vi "slow_control_2_10.vi"() -> ()   [LabVIEW 2018]
uses:
  4623b864-5764-45c6-9cb2-3e18237880ca.vi
  fa57f61f-0bb9-49ac-92eb-fcb40add4dbb.vi
  499f9cf5-7b15-41ea-951a-8da9be12721d.vi
  <vilib>/DAQmx/read.llb/DAQmx Read (Analog 1D DBL NChan 1Samp).vi
  ffb0d1b3-ef19-4e2e-b36e-7277177ef4b3.vi
  9a1acc8a-69db-4048-9e4c-bb07d66d2422.vi
  <vilib>/DAQmx/create/channels.llb/DAQmx Create Channel (AI-Voltage-Basic).vi
  <vilib>/DAQmx/create/channels.llb/DAQmx Create Channel (AI-Current-Basic).vi
  <vilib>/DAQmx/create/channels.llb/DAQmx Create Channel (AI-Temperature-RTD).vi
  <vilib>/DAQmx/miscellaneous.llb/DAQmx Fill In Error Info.vi
  <vilib>/Utility/file.llb/Read Delimited Spreadsheet (string).vi
  <instrlib>/Lake Shore 335/Lake Shore 335.lvlib
  <instrlib>/CAEN PSM/CAEN PSM.lvlib
  <resource>/objmgr/daqmx.rc
panel:
  out "Heater":dbl
  out "Coldhead":dbl
  out "Cycle number":i32
  out "Alarm state":bool
  out "Timestamp last \nmeasured (UPS)":timestamp
  out "Auto-clear":bool
  in  "Auto-clear data?":bool
  in  "Clear data":bool
  in  "Clear data every N cycles":dbl
  in  "N samples":i32=30
  out "Average Flow (SLPM)":dbl caption="Flow (SLPM)"
  out "CAEN Ch. Names":string[](array[string])
  in  "Cycles to execute":dbl=5.0 format="%#_13g"
  out "Detector Pressure":dbl
  in  "N samples":i32=20
  in  "Allows tabs on \nfront panel":T1(tab)
  in  "Specify up to six temperature sensors inside \nthe detector, separated with a comma.\nNumbers only, single commas!":string="10,11,12,13,14,15"
  out "Valid example:":string="11,12, 13, 15 ,14 "
  in  "Anode ch.":enum16{"1", "2", "3", "4"}(ring)=enum."3"
  in  "CAEN unit selector":enum16{"CAEN 1", "CAEN 2"}(ring)
  in  "Multipliers":dbl[](array[numeric])=[1.0, 1.0, 1.0, 1.0, 1.0, 1.0, 1.0, 1.0]
  in  "Offsets\nsubtracted":dbl[](array[numeric])=[0.0, 0.0, 0.0, 0.0, 0.0, 0.0, 0.0, 0.0]
  in  "Channel Names (9207, ai8:15)":string[](array[string])=["i0", "i1", "i2", "i3", "i4", "i5", "i6", "i7"] caption="\"Other\""
  in  "Flow meter input:":u16(ring)=3 items=["v0", "v1", "v2", "v3", "v4", "v5", "v6", "v7"]
  in  "Detector pressure input:":u16(ring) items=["v0", "v1", "v2", "v3", "v4", "v5", "v6", "v7"]
  in  "Channel Names (9207, ai0:7)":string[](array[string])=["v0", "v1", "v2", "v3", "v4", "v5", "v6", "v7"] caption="\"Other\""
  in  "Multipliers":dbl[](array[numeric])=[1.0, 1.0, 1.0, 1.0, 1.0, 1.0, 1.0, 1.0]
  in  "Offsets\nsubtracted":dbl[](array[numeric])=[0.0, 0.0, 0.0, 0.0, 0.0, 0.0, 0.0, 0.0]
  in  "Voltage channels":tag[](array[tag])=["9207/ai0", "9207/ai1", "9207/ai2", "9207/ai3", "9207/ai4", "9207/ai5", "9207/ai6", "9207/ai7"]
  in  "COM-port CAEN 1":refnum<visa-resource-name>
  in  "COM-port CAEN 2":refnum<visa-resource-name>
  out "LakeShore readings 2":dbl[](array[numeric])
  in  "Run lakeshore?":bool
  in  "ID Query":bool
  in  "COM-port LakeShore":refnum<visa-resource-name>
  in  "PID settings":cluster{"P":dbl, "I":dbl, "D":dbl}={"P"=50.0, "I"=20.0, "D"=120.0}
  in  "Setpoint (°C)":dbl=-100.0 format="%.1f"
  in  "Heater range":u16(ring) items=["Off", "Low (On)", "Medium", "High"]
  in  "Current channels":tag[](array[tag])=["9207/ai8", "9207/ai9", "9207/ai10", "9207/ai11", "9207/ai12", "9207/ai13", "9207/ai14", "9207/ai15"]
  in  "Channel Names (CAEN)":string[](array[string])=["PMT 1", "PMT 2", "Anode", "Cathode", "Top gate", "Bottom gate", "Other 1", "Other 2"]
  in  "RTD Type":i32(ring)=12481 items=["Pt3750"=12481, "Pt3851"=10071, "Pt3911"=12482, "Pt3916"=10069, "Pt3920"=10053, "Pt3928"=12483, "Custom"=10137]
  in  "Module 1 channels (slot 1)":tag[](array[tag])
  in  "Current Excitation Source":i32(ring)=10200 items=["Internal"=10200, "External"=10167, "None"=10230]
  in  "Resistance Configuration":i32(ring)=3 items=["2-Wire"=2, "3-Wire"=3, "4-Wire"=4]
  in  "R (T = 0°C):":dbl=100.0
  in  "B":dbl
  in  "A":dbl
  in  "C":dbl
  in  "Module 2 channels (slot 2)":tag[](array[tag])
  in  "Shut off heater \nif Alarm is active":bool=TRUE
  in  "Re-save headers":bool
  out "Det. T.":i32[](array[numeric])
  out "9207 (V; A) Converted":dbl[](array[numeric])
  out "9216 #1 (°C)":dbl[](array[numeric])
  out "9216 #2 (°C)":dbl[](array[numeric])
  out "Raw readouts (V, mA)":dbl[](array[numeric]) format="%0.2f"
  out "Det.P input #":i32
  out "Flow input #":i32
  out "Temperatures":dbl[](array[numeric]) format="%0.2f"
  in  "\"Sound\" alarm":bool
  in  "Sound alarm\nFrequency (Hz)":dbl=1680.0
  in  "Send status email now":bool
  out "Email error":i32
  out "source":string
  in  "Number of Bonus lines":i32=1
  out "Names (optional)":string[](array[string])
  in  "Send daily email?":bool=TRUE
  in  "Phone numbers":string[](array[string])
  out "Alarm (or test) message":string
  in  "Alarm\nMaster switch":bool
  in  "Repeat Alarm SMS\nevery N minutes":dbl=15.0
  in  "Test alarm":bool
  out "Warning":bool
  in  "UPS":bool
  in  "UPS Voltage \nLower Threshold":dbl=220.0
  out "String 6":string
  out "String 5":string
  out "String 4":string
  out "String 3":string
  out "String 2":string
  out "String":string
  out "NI mod 2&3 status":bool
  in  "NI mod 2&3":bool
  in  "NI mod 1":bool
  in  "CAEN 2":bool
  in  "CAEN 1":bool
  in  "LakeShore":bool
  out "Det. P. warning":bool
  out "Boolean 6":bool
  out "Boolean 5":bool
  out "Boolean 4":bool
  out "Boolean 3":bool
  out "Boolean 2":bool
  out "Boolean":bool
  in  "T 6":bool
  in  "T 5":bool
  in  "T 4":bool
  in  "T 3":bool
  in  "T 2":bool
  in  "T 1":bool
  in  "Detector Pressure":bool
  in  "Overpressure threshold":dbl
  in  "Underpressure threshold":dbl
  out "Comm. status":bool
  in  "High Temp threshold":dbl format="%#_13g"
  in  "Low Temp threshold":dbl format="%#_13g"
  out "LakeShore status":bool
  out "NI mod1 (P) status":bool
  out "CAEN 1 status":bool
  out "CAEN 2 status":bool
  out "Initialization status":bool
  out "Minimum input voltage measured":dbl
  out "Alarm active 2":bool
  out "SMS error":string
  out "Status email preview":string
  in  "Send status email at time:":string="14:00"
  in  "Email Addresses":string[](array[string])
  in  "return address":string="xamsups@gmail.com"
  in  "Ignore Initialization Errors":bool=TRUE caption="Ignore init. errors?"
  out "9207 (ai 8:15, Amperes)":cluster{timestamp[], dbl[]}[](graph)
  in  "Temperature channel selector":u16(ring)=10 items=["10"=10, "11"=11, "12"=12, "13"=13, "14"=14, "15"=15, "Average"=666]
  out "Heater power (%)":cluster{timestamp[], dbl[]}[](graph)
  out "Flow (SLPM)":cluster{timestamp[], dbl[]}[](graph)
  out "9207 (ai 0:7, Volts)":cluster{timestamp[], dbl[]}[](graph)
  out "Phase Diagram":cluster{"X":dbl, "Y":dbl}[](graph)
  out "Temperature (ai 0:15, °C)":cluster{timestamp[], dbl[]}[](graph)
  in  "Pause?":bool
  out "Integrated Flow (SL)":dbl
  in  "Reset?":bool
  out "LakeShore readings":dbl[](array[numeric])
  out "Temp A":dbl
  out "Temp B":dbl
  in  "Temperature Channel Selector":u16(ring) items=["10"=10, "11"=11, "12"=12, "13"=13, "14"=14, "15"=15]
  out "Historical Large Phase Diagram":cluster{dbl[], dbl[]}[](graph)
  out "Large Phase Diagram":cluster{"X":dbl, "Y":dbl}[](graph)
  in  "Temperature Channel Selector":u16(ring)=666 items=["10"=10, "11"=11, "12"=12, "13"=13, "14"=14, "15"=15, "Average"=666]
  in  "Scale.Range:Minimum 8":dbl
  in  "Scale.Range:Maximum 8":dbl=4000.0
  in  "Scale.Range:Minimum 7":dbl
  in  "Scale.Range:Maximum 7":dbl=4000.0
  in  "Scale.Range:Minimum 6":dbl=-3000.0
  in  "Scale.Range:Maximum 6":dbl
  in  "Scale.Range:Minimum 5":dbl
  in  "Scale.Range:Maximum 5":dbl=3000.0
  in  "Scale.Range:Minimum 4":dbl=-5000.0
  in  "Scale.Range:Maximum 4":dbl
  in  "Scale.Range:Maximum 3":dbl=4000.0
  in  "Scale.Range:Minimum 3":dbl
  in  "Scale.Range:Maximum 2":dbl=1000.0
  in  "Scale.Range:Minimum 2":dbl
  out "CAEN 1.1":dbl(knob) scale=0.0..1000.0
  out "CAEN 1.1":string
  in  "Scale.Range:Maximum":dbl=1000.0
  in  "Scale.Range:Minimum":dbl
  out "CAEN 2.3 2":string
  out "CAEN 2.2 2":string
  out "Channel Names":string[](array[string])
  out "CAEN 2.3":dbl(knob) scale=0.0..4000.0
  out "CAEN 2.2":dbl(knob) scale=0.0..4000.0
  out "CAEN 2.1":string
  out "CAEN 2.0":string
  out "CAEN 1.3":string
  out "CAEN 1.2":string
  out "CAEN 1.0":string
  out "Channel Names":string[](array[string])
  in  "Set to zero":bool
  out "CAEN 2.1":dbl(knob)
  out "CAEN 2.0":dbl(knob) scale=0.0..3000.0
  in  "Apply Voltage":bool
  in  "VSet (V)":dbl[](array[numeric])
  in  "IMax (uA)":dbl[](array[numeric])
  in  "VMax (V)":dbl[](array[numeric])
  out "CAEN 1.3":dbl(knob)
  out "CAEN 1.2":dbl(knob) scale=0.0..4000.0
  out "CAEN 1.0":dbl(knob) scale=0.0..1000.0
  out "Vmon (V)":dbl[](array[numeric])
  out "IMon (uA)":dbl[](array[numeric])
  in  "Read CAEN units \nevery N cycles":i16=120
  in  "Reset anode\nperiodically?":bool
  in  "Kill every Y minutes":i32=10
  in  "Keep off for X seconds":i32=10
  out "?":bool
  out "Killed":bool
  out "Restarted":bool
  out "Anode timers":timestamp[](array[timestamp])
  out "Seconds until \nanode autokill":dbl format="%.2g"
  out "Seconds until \nanode reset":dbl format="%.2g"
  in  "Kill voltage":bool
  in  "stop":bool
  out "Voltages":dbl[](array[numeric])
  out "Started up?":bool
  out "TOBA appended":dbl[][](array[numeric])
  in  "Read T every N cycles":i32=2
  out "Time until next cycle":dbl format="%.3g"
  in  "Time per cycle (s)":i32=2 caption="Time Target (s)"
  # "<- Proof of concept for New/Old T + New P"
  # "Moving averages"
  # "NI 9216 Temperature settings"
  # "CAEN settings"
  # "NI 9207 Voltage settings"
  # "If RTD type is custom,\nspecify the Callendar-\nVan Dusen parameters"
  # "Anode connected to:"
  # "Channel:"
  # "NI 9207 Current settings"
  # "Lakeshore settings"
  # "Brum hier"
  # "Gain (P) (XX.X)"
  # "Reset (I) (XX.X)"
  # "Rate (D) (X.X%)"
  # "Alarm indicators and arms"
  # "Detector Thresholds"
  # "Daily status email"
  # "SMS and sound alarm"
  # "Alarm conditions"
  # "Temperature channels:"
  # "Uninterruptable Power Supply"
  # "Data"
  # "Scale:"
  # "to"
  # "to"
  # "Scale:"
  # "Time of last reset"
  # "Time of last reactivation"
  # "to"
  # "Scale:"
  # "to"
  # "Scale:"
  # "Settings"
  # "Scale:"
  # "to"
  # "Scale:"
  # "to"
  # "Scale:"
  # "to"
  # "to"
  # "Scale:"
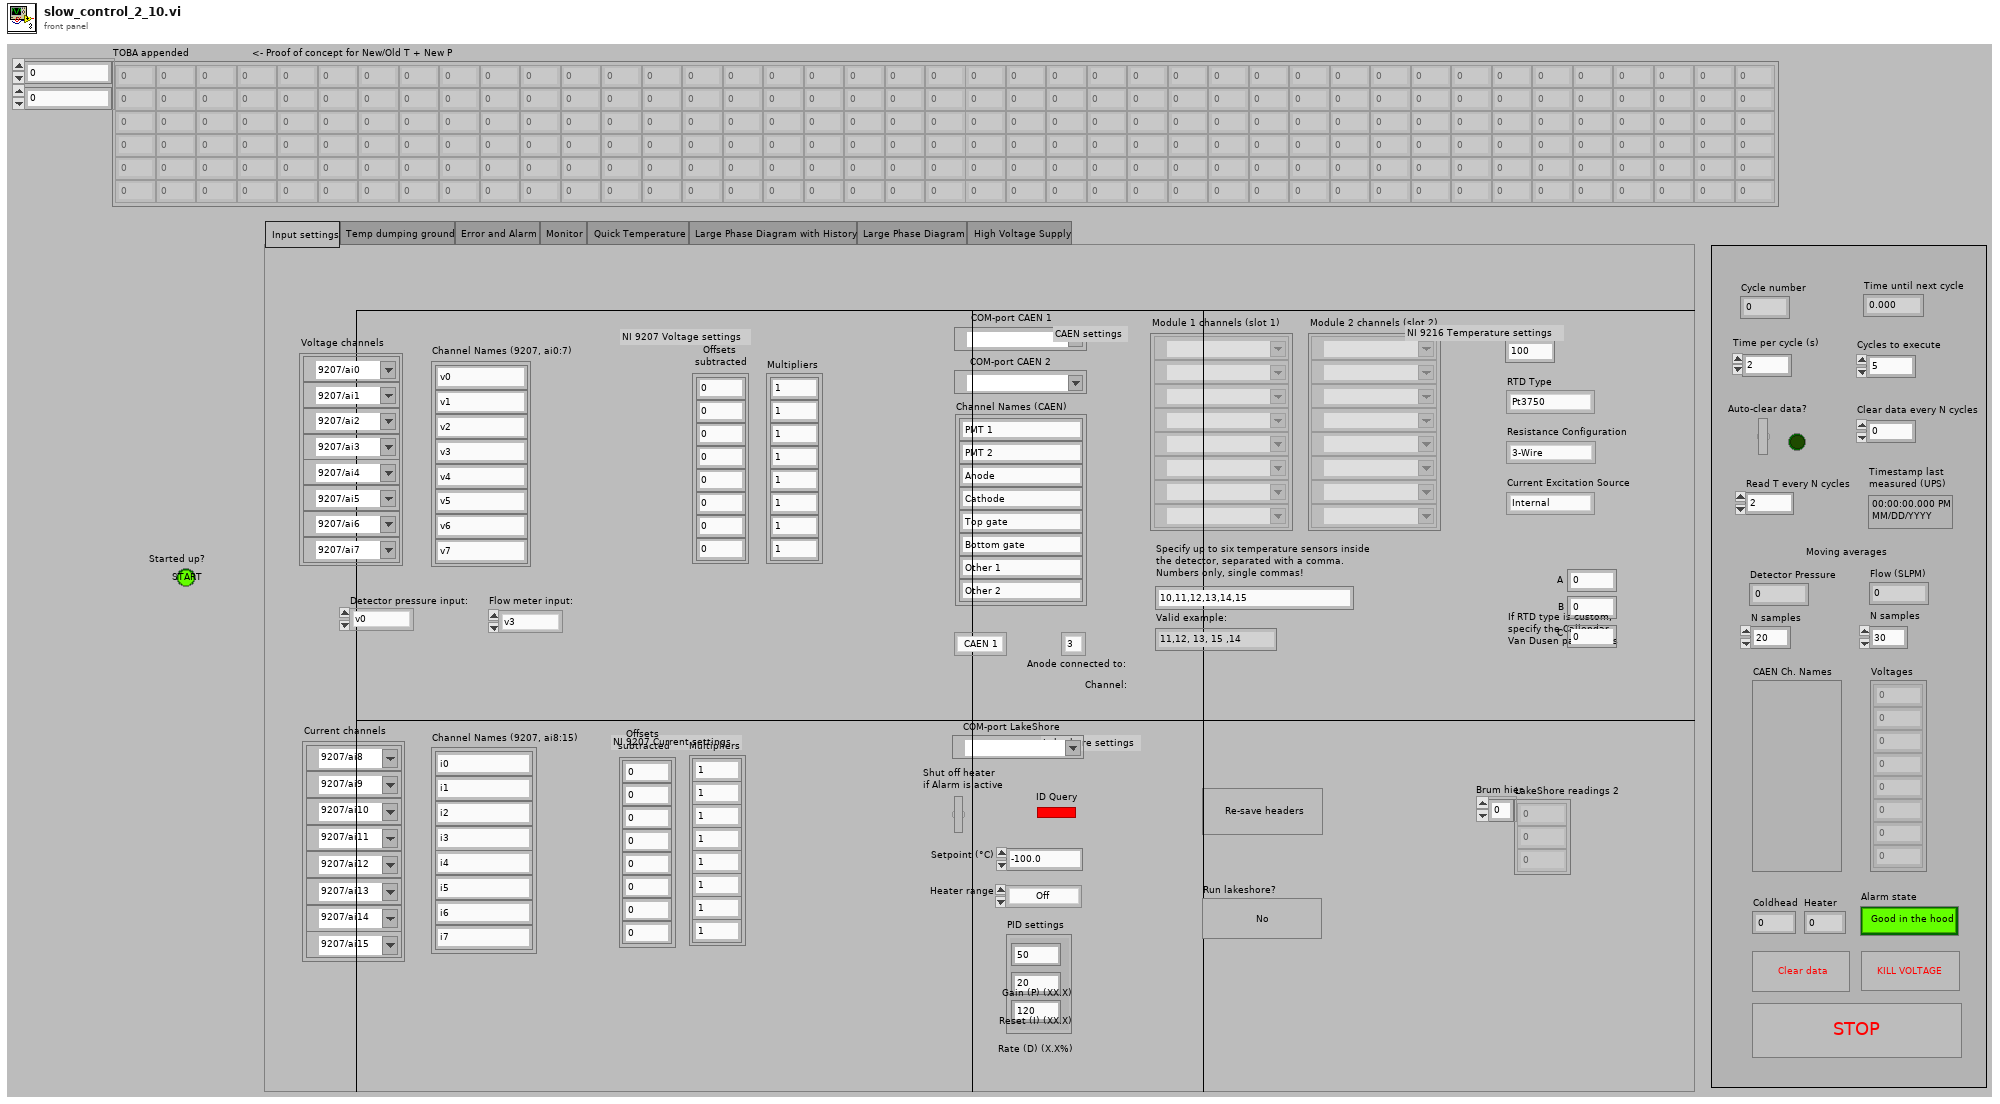
[diagram p1: front panel]
types:
  T1 = enum32{"Input settings", "Temp dumping ground", "Error and Alarm", "Monitor", "Quick Temperature", "Large Phase Diagram with History", "Large Phase Diagram", "High Voltage Supply"}
  T2 = cluster{"Baud Rate":u32, "Parity":u16, "Data Bits":u16, "Stop Bits":u16, "Flow Control":u16}
  T3 = cluster{"VISA resource name out":refnum<visa-resource-name>, "error out":errorcluster}
  T4 = cluster{"task out":refnum<k21>, "error out":errorcluster}
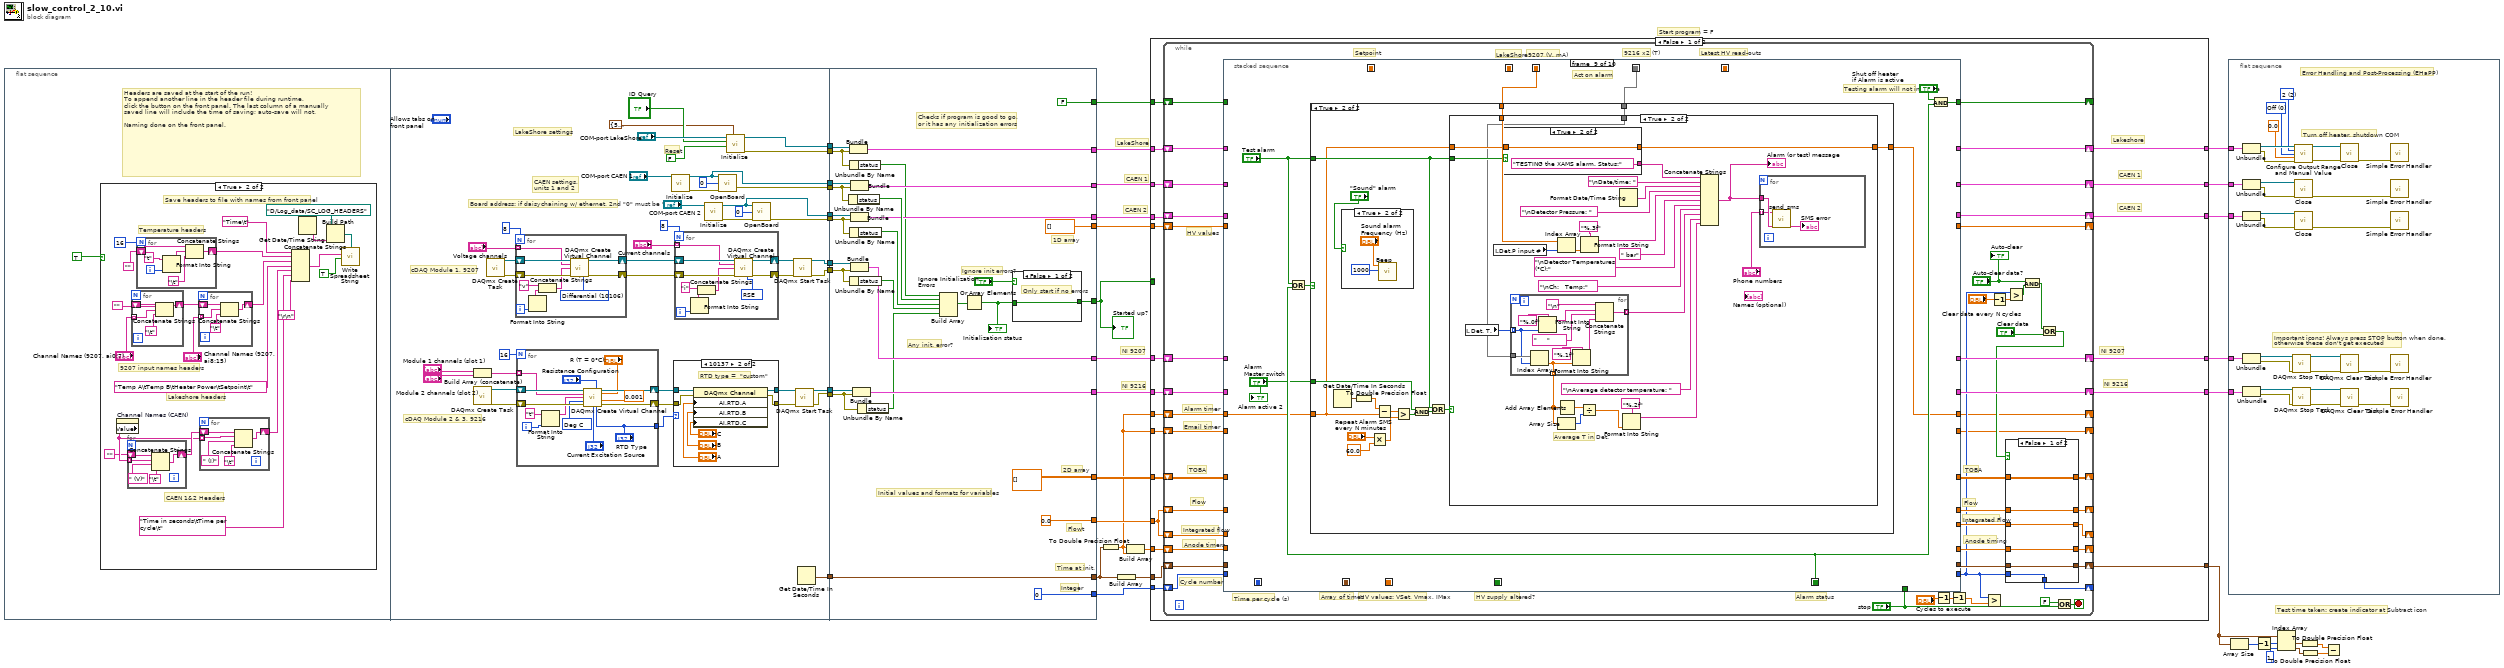
[diagram p0: block diagram]
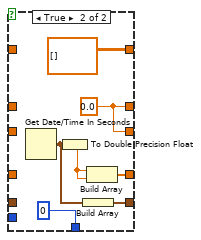
[diagram p2: hidden frame]
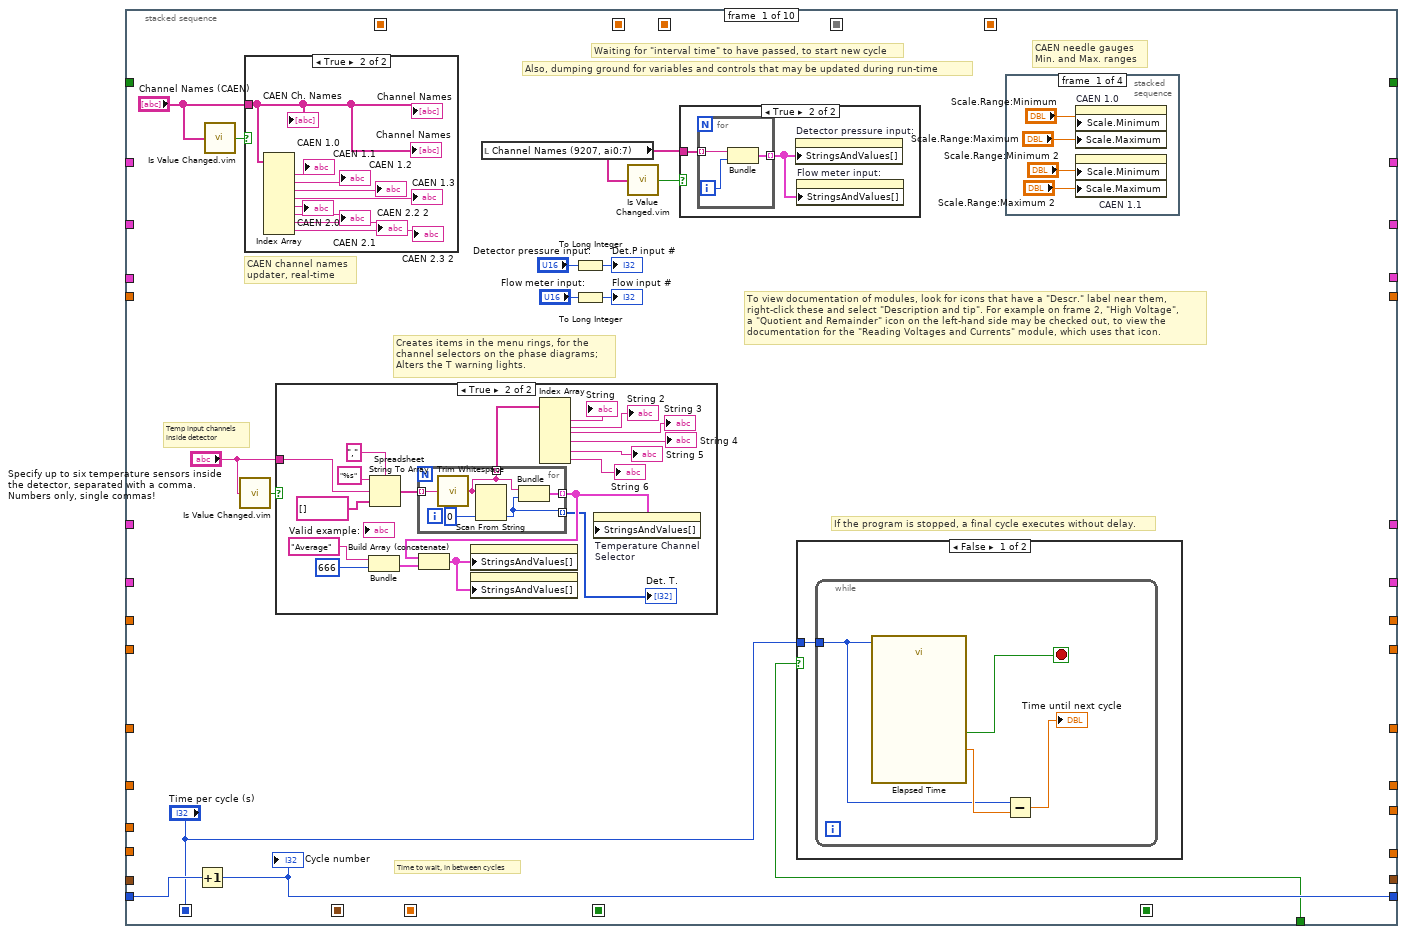
[diagram p3: hidden frame]
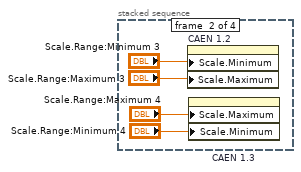
[diagram p7: hidden frame]
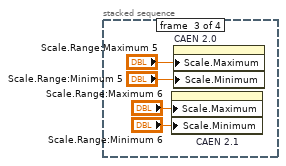
[diagram p8: hidden frame]
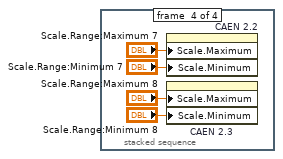
[diagram p9: hidden frame]
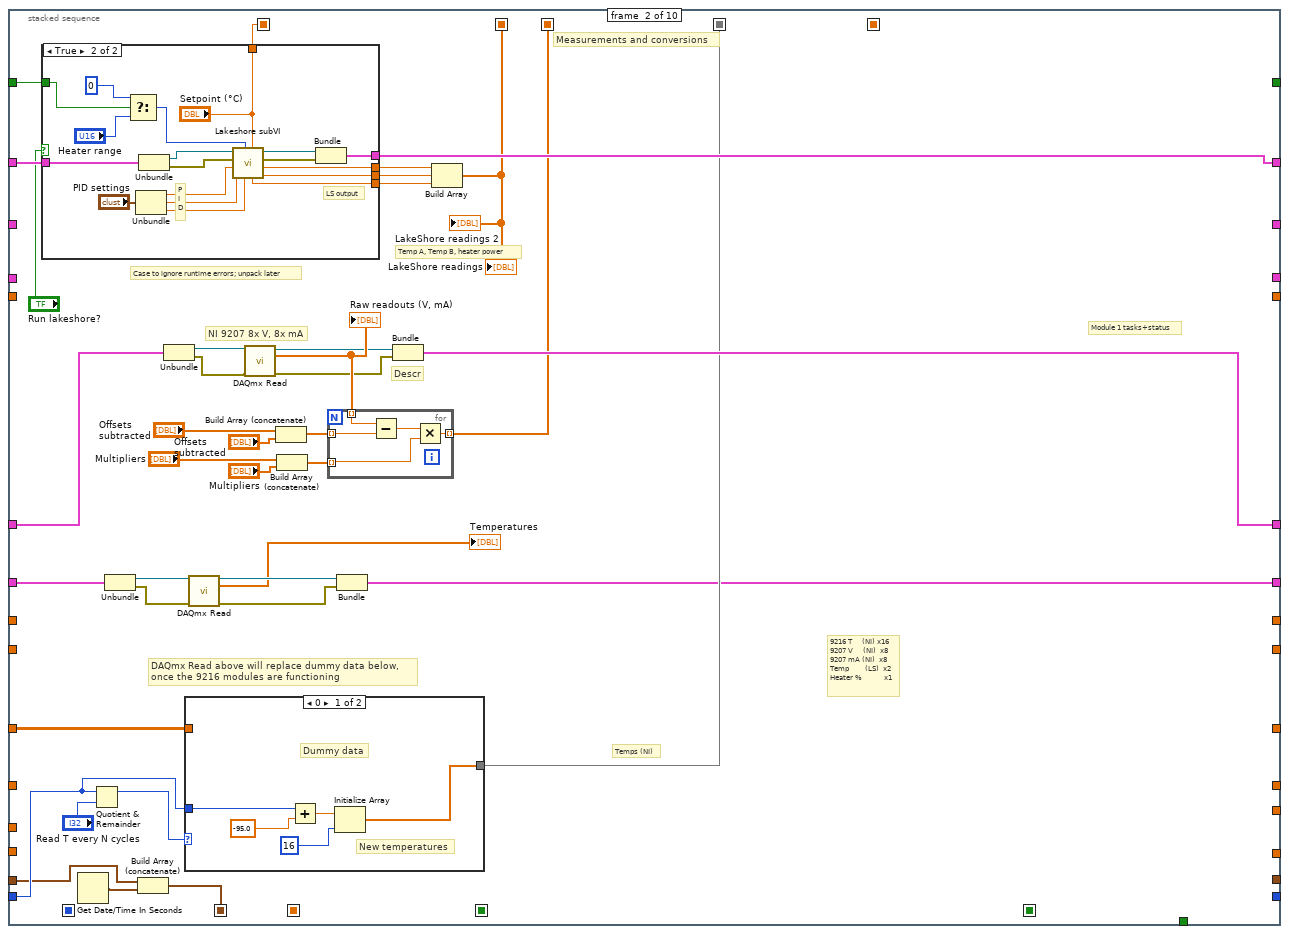
[diagram p11: hidden frame]
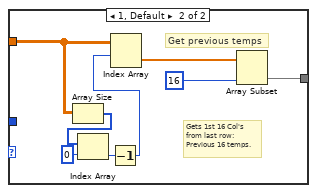
[diagram p12: hidden frame]
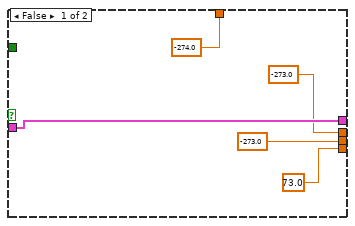
[diagram p13: hidden frame]
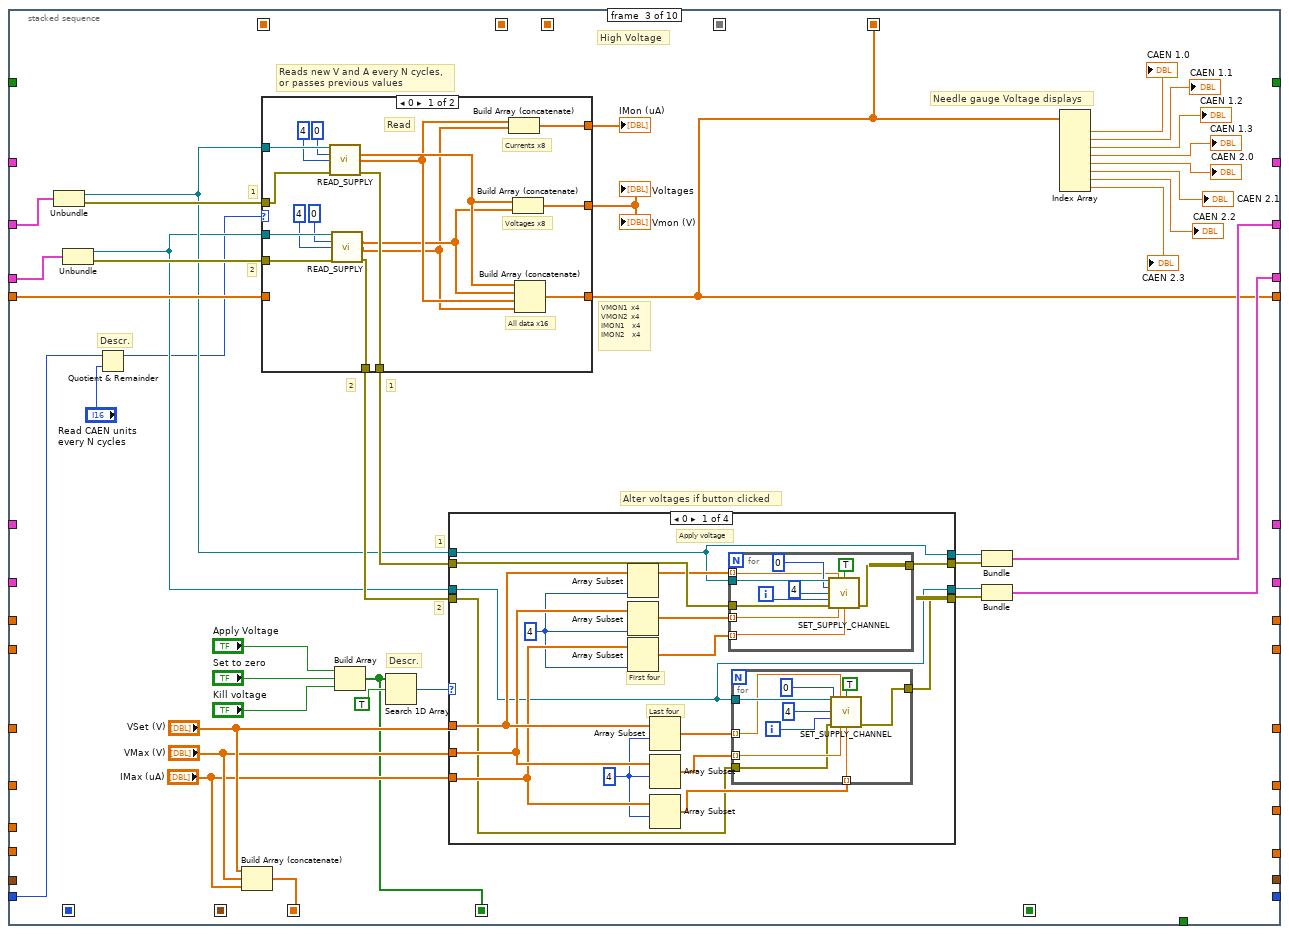
[diagram p14: hidden frame]
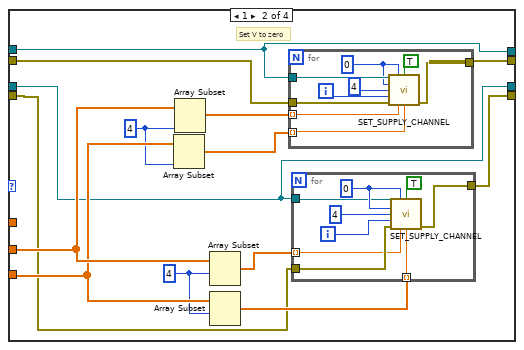
[diagram p15: hidden frame]
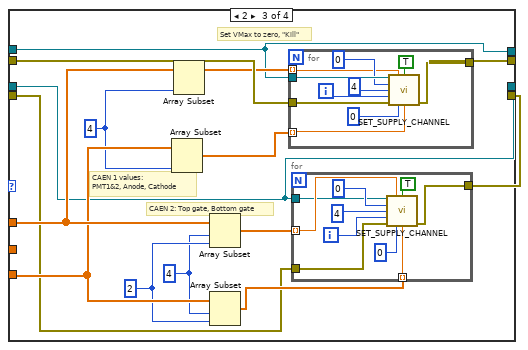
[diagram p16: hidden frame]
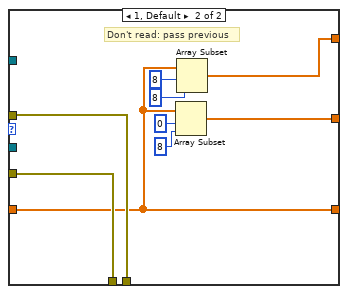
[diagram p18: hidden frame]
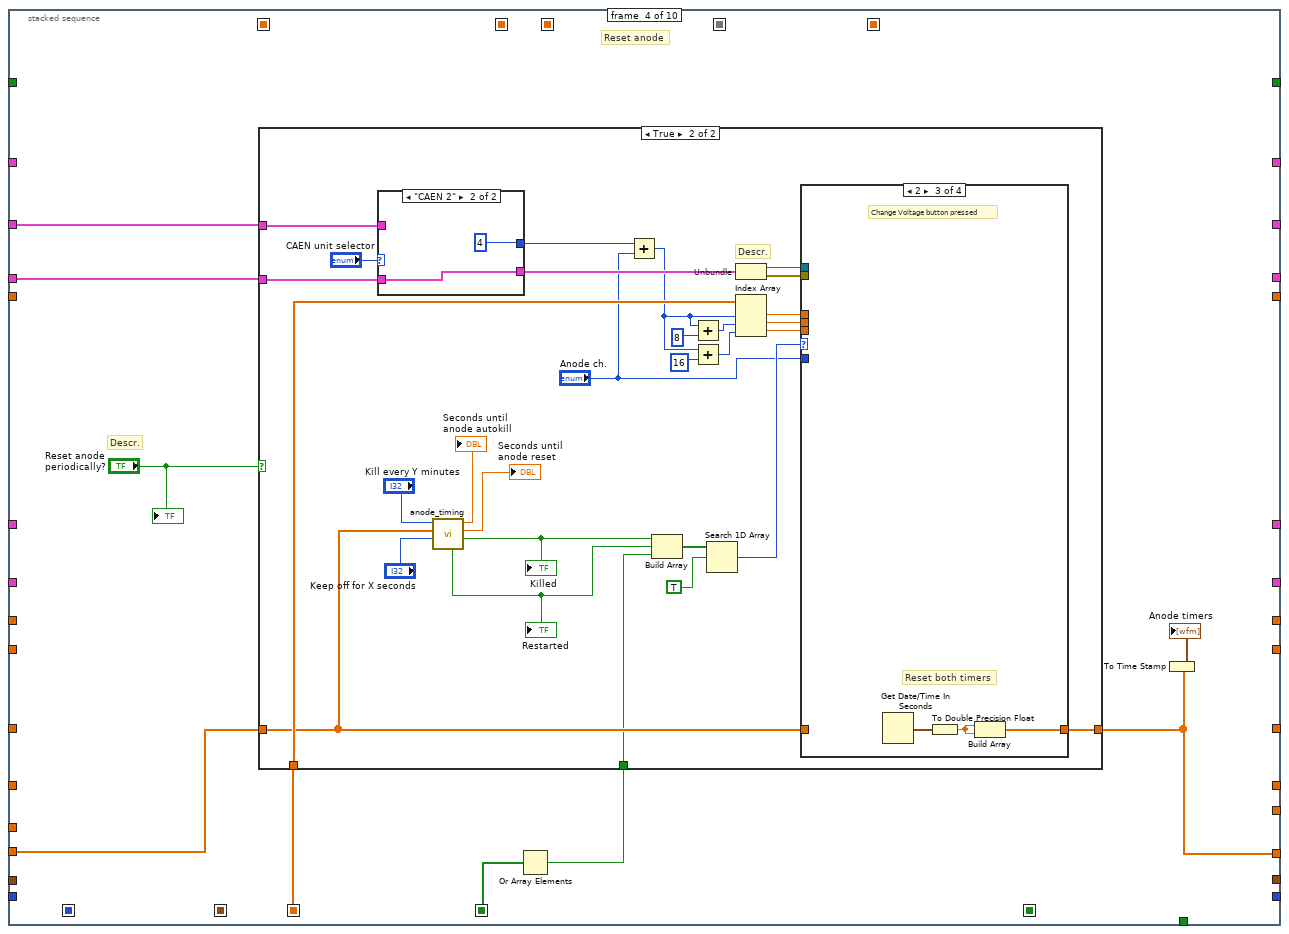
[diagram p19: hidden frame]
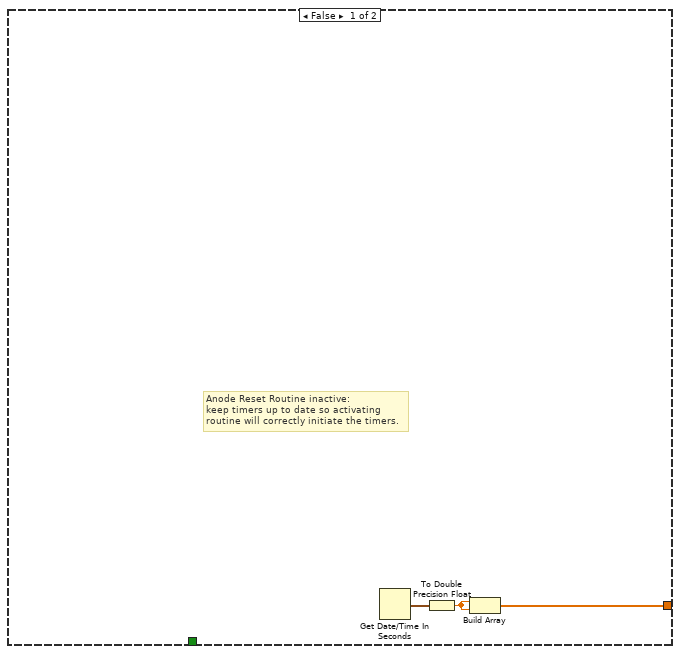
[diagram p20: hidden frame]
diagram:
  # "NI 9216"
  # "Test time taken: create indicator at Subtract icon"
  # "NI 9207"
  # "Start program = F"
  # "CAEN 2"
  # "CAEN 1"
  # "LakeShore"
  n1 = flat-sequence {
    tunnel: [w124] -> w39
    tunnel: [w123] -> w38
    tunnel: [w111] -> w37
    tunnel: [w120] -> w36
    tunnel: [w101] -> w35
    tunnel: [w119] -> w30
    tunnel: [w115] -> w22
    tunnel: [w114] -> w21
    tunnel: [w102] -> w13
    tunnel: [w96] -> w5
    tunnel: [w95] -> w4
    tunnel: w39 -> [w197]
    tunnel: w38 -> [w196]
    tunnel: w37 -> [w194]
    tunnel: w36 -> [w193]
    tunnel: w35 -> [w183]
    tunnel: [w198] -> w19
    tunnel: [0.0] -> w18
    tunnel: [dbl[] []] -> w34
    tunnel: [dbl[][] []] -> w6
    tunnel: [0] -> w33
    tunnel: [w195] -> w32
    tunnel: [w192] -> w31
    tunnel: [w191] -> w17
    tunnel: w30 -> [w191]
    tunnel: w22 -> [w189]
    tunnel: w21 -> [w188]
    tunnel: [w187] -> w20
    tunnel: [FALSE] -> w14
    tunnel: w13 -> [w184]
    tunnel: [w182] -> w12
    tunnel: w5 -> [w175]
    tunnel: w4 -> [w174]
    tunnel: [w173] -> w3
    frame #0 {
      # "Headers are saved at the start of the run!\nTo append another line in the header file during runtime,\nclick the button on the front panel. The last column of a manually\nsaved line will include the time of saving; auto-save will not.\n\nNaming done on the front panel."
      n2 = case shown="True" TRUE {
        frame False {
        }
        frame True {
          # "CAEN 1&2 Headers"
          # "Lakeshore headers"
          # "9207 input names headers"
          # "Temperature headers"
          # "Save headers to file with names from front panel"
          n3 = property on="Channel Names (CAEN)" class="Arr (strict)"() -> ("Value"=w46:string[])  [unwired: 2 in, 2 out]
          n4 = for {
            tunnel: w46 -> [w70] mode=indexing
            shift-right: [w68] -> w47
            shift-left: "" -> [w67]
            n5 = Concatenate Strings(w67, w70, " (V)", "\t") -> (w68:string)
          }
          n6 = for {
            shift-right: [w78] -> w50
            shift-left: "" -> [w79]
            tunnel: "Channel Names (9207, ai0:7)" -> [w76] mode=indexing
            n7 = Concatenate Strings(w79, w76, "\t") -> (w78:string)
          }
          n8 = for {
            N: 16 -> [_]
            shift-right: [w80] -> w53
            shift-left: "" -> [w81]
            i -> [w85]
            n9 = Format Into String(initial string="t", w85) -> (resulting string=w83:string)  [unwired: 2 in, 1 out]
            n10 = Concatenate Strings(w81, w83, "\t") -> (w80:string)
          }
          n11 = for {
            shift-right: [w73] -> w49
            shift-left: w50 -> [w75]
            tunnel: "Channel Names (9207, ai8:15)" -> [w72] mode=indexing
            n12 = Concatenate Strings(w75, w72, "\t") -> (w73:string)
          }
          n13 = for {
            shift-right: [w63] -> w45
            shift-left: w47 -> [w64]
            tunnel: w46 -> [w62] mode=indexing
            n14 = Concatenate Strings(w64, w62, " (I)", "\t") -> (w63:string)
          }
          n15 = Concatenate Strings("Time\t", w53, w49, "Temp A\tTemp B\tHeater Power\tSetpoint\t", w45, "Time in seconds\tTime per cycle\t", "\r\n") -> (w52:string)
          n16 = Get Date/Time String() -> (date string=w56:string)  [unwired: 3 in, 1 out]
          n17 = Build Path(base path=path "D:/Log_data/SC_LOG_HEADERS" ("file path (dialog if empty)"), name or relative path=w56) -> (appended path=w57:path)
          n18 = call <vilib>:"Write Spreadsheet String.vi"("append to file? (new file:F)"=TRUE, "spreadsheet string"=w52, "file path (dialog if empty)"=w57) -> ()  [unwired: 7 in, 2 out]
        }
      }
    }
    frame #1 {
      # "cDAQ Module 2 & 3, 9216"
      # "cDAQ Module 1, 9207"
      # "Board address: if daisychaining w/ ethernet, 2nd \"0\" must be \"1\""
      # "CAEN settings,\nunits 1 and 2"
      # "Reset"
      # "LakeShore settings"
      n19 = call <vilib>:"DAQmx Create Task.vi"() -> ("task out"=w94:refnum<k21>, "error out"=w97:errorcluster)  [unwired: 14 in]
      n20 = Build Array (concatenate)("Module 1 channels (slot 1)", "Module 2 channels (slot 2)") -> (w91:tag[])
      n21 = call <vilib>:"DAQmx Create Task.vi"() -> ("task out"=w110:refnum<k21>, "error out"=w109:errorcluster)  [unwired: 14 in]
      n22 = for {
        N: 8 -> [_]
        shift-right: [w166] -> w106
        shift-left: w110 -> [w165]
        shift-right: [w167] -> w105
        shift-left: w109 -> [w163]
        tunnel: "Voltage channels" -> [w164] mode=indexing
        i -> [w169]
        w161 = 10106 items=["Default"=-1, "RSE"=10083, "NRSE"=10078, "Differential"=10106, "Pseudodifferential"=12529] ("input terminal configuration")
        n23 = Format Into String(w169) -> (resulting string=w168:string)  [unwired: 3 in, 1 out]
        n24 = Concatenate Strings("v" ("string"), w168) -> (w162:string)
        n25 = call-poly <vilib>:"DAQmx Create Virtual Channel.vi"("task in"=w165, "input terminal configuration"=w161, "physical channels"=w164, "name to assign"=w162, "error in"=w163) -> ("task out"=w166:refnum<k21>, "error out"=w167:errorcluster)  [unwired: 9 in]
      }
      n26 = for {
        N: 16 -> [_]
        shift-right: [w147] -> w90
        shift-left: w94 -> [w150]
        shift-right: [w148] -> w89
        shift-left: w97 -> [w149]
        tunnel: w91 -> [w146] mode=indexing
        tunnel: ["RTD Type"] -> w86
        i -> [w144]
        w141 = 10143 items=["Deg C"=10143, "Deg F"=10144, "Kelvins"=10325, "Deg R"=10145, "From Custom Scale"=10065] ("units")
        n27 = Format Into String(initial string="t", w144) -> (resulting string=w143:string)  [unwired: 2 in, 1 out]
        n28 = call-poly <vilib>:"DAQmx Create Virtual Channel.vi"("task in"=w150, "resistance configuration"="Resistance Configuration", "physical channels"=w146, "r0"="R (T = 0°C):", "name to assign"=w143, "units"=w141, "current excitation value"=0.001, "error in"=w149, "current excitation source"="Current Excitation Source", "rtd type"="RTD Type") -> ("task out"=w147:refnum<k21>, "error out"=w148:errorcluster)  [unwired: 4 in]
      }
      n29 = call <instrlib>:"Initialize.vi"("VISA resource name"="COM-port CAEN 1") -> ("error out"=w121:errorcluster, "VISA resource name out"=w111:refnum<visa-resource-name>)  [unwired: 9 in]
      n30 = case shown="10137" w86 {
        tunnel: w90 -> [w129 w133]
        tunnel: w89 -> [w128 w132]
        tunnel: [w129 w131] -> w88
        tunnel: [w128 w130] -> w87
        frame 0, Default {
          # "Don't need to specify the A, B, C\nvalues if RTD type is not \"custom\""
        }
        frame 10137 {
          # "RTD type =  \"custom\""
          n31 = property class="DAQmx Channel"(reference=w133, error in=w132, "AI.RTD.A"="A", "AI.RTD.B"="B", "AI.RTD.C"="C") -> (reference out=w131:refnum<k21>, error out=w130:errorcluster)
        }
      }
      n32 = for {
        N: 8 -> [_]
        shift-right: [w152] -> w103
        shift-left: w106 -> [w159]
        shift-right: [w151] -> w104
        shift-left: w105 -> [w158]
        tunnel: "Current channels" -> [w157] mode=indexing
        i -> [w156]
        w160 = 10083 items=["default"=-1, "RSE"=10083, "NRSE"=10078, "Differential"=10106, "Pseudodifferential"=12529] ("input terminal configuration")
        n33 = Format Into String(w156) -> (resulting string=w154:string)  [unwired: 3 in, 1 out]
        n34 = Concatenate Strings("i", w154) -> (w153:string)
        n35 = call-poly <vilib>:"DAQmx Create Virtual Channel.vi"("task in"=w159, "input terminal configuration"=w160, "physical channels"=w157, "name to assign"=w153, "error in"=w158) -> ("task out"=w152:refnum<k21>, "error out"=w151:errorcluster)  [unwired: 9 in]
      }
      n36 = call <instrlib>:"Initialize.vi"("VISA resource name"="COM-port CAEN 2") -> ("error out"=w116:errorcluster, "VISA resource name out"=w115:refnum<visa-resource-name>)  [unwired: 9 in]
      n37 = call <instrlib>:"OpenBoard.vi"("error in (no error)"=w121, "Board Address"=0, "VISA resource name"=w111) -> ("error out"=w120:errorcluster)  [unwired: 7 in, 1 out]
      n38 = call <instrlib>:"Initialize.vi"("Serial Configuration"=T2 {"Baud Rate"=57600, "Parity"=1, "Data Bits"=7, "Stop Bits"=10, "Flow Control"=0}, "Reset (True)"=FALSE ("Reset (LakeShore)"), "ID Query (True)"="ID Query", "VISA resource name"="COM-port LakeShore") -> ("error out"=w123:errorcluster, "VISA resource name out"=w124:refnum<visa-resource-name>)  [unwired: 6 in]
      n39 = call <instrlib>:"OpenBoard.vi"("error in (no error)"=w116, "Board Address"=u8 0, "VISA resource name"=w115) -> ("error out"=w114:errorcluster)  [unwired: 7 in, 1 out]
      n40 = call <vilib>:"DAQmx Start Task.vi"("task/channels in"=w103, "error in"=w104) -> ("task out"=w102:refnum<k21>, "error out"=w101:errorcluster)  [unwired: 12 in]
      n41 = call <vilib>:"DAQmx Start Task.vi"("task/channels in"=w88, "error in"=w87) -> ("task out"=w96:refnum<k21>, "error out"=w95:errorcluster)  [unwired: 12 in]
      n42 = Get Date/Time In Seconds() -> (seconds since 1Jan1904=w119:timestamp)
    }
    frame #2 {
      # "1D array"
      # "Initial values and formats for variables"
      # "Time at init."
      # "Integer"
      # "2D array"
      # "Flowt"
      # "Checks if program is good to go,\nor it has any initialization errors"
      # "Ignore init errors?"
      # "Any init. error?"
      n43 = Unbundle By Name(w193) -> ("status"=w199:bool)
      n44 = Unbundle By Name(w196) -> ("status"=w176:bool)
      n45 = Bundle("VISA resource name out"=w197, "error out"=w196) -> (w195:T3)  [unwired: 1 in]
      n46 = Unbundle By Name(w188) -> ("status"=w190:bool)
      n47 = Unbundle By Name(w183) -> ("status"=w177:bool)
      n48 = Bundle("VISA resource name out"=w189, "error out"=w188) -> (w187:T3)  [unwired: 1 in]
      n49 = Bundle("task out"=w184, "error out"=w183) -> (w182:T4)  [unwired: 1 in]
      n50 = Bundle("VISA resource name out"=w194, "error out"=w193) -> (w192:T3)  [unwired: 1 in]
      n51 = Bundle("task out"=w175, "error out"=w174) -> (w173:T4)  [unwired: 1 in]
      n52 = Unbundle By Name(w174) -> ("status"=w172:bool)
      n53 = Build Array(w176, w199, w177, w190, w172) -> (w200:bool[])
      n54 = Or Array Elements(Boolean array=w200) -> (logical OR=w171:bool)
      "Initialization status" <- w171
      n55 = case shown="False" "Ignore Initialization Errors" {
        tunnel: [w201 FALSE] -> w198
        tunnel: w171 -> [w201 _]
        frame False {
          # "Only start if no errors"
        }
        frame True {
          # "Always start program"
        }
      }
    }
  }
  n56 = To Double Precision Float(number=w17) -> (double precision float=w1:dbl)
  n57 = Build Array(w17) -> (w29:timestamp[])
  n58 = Build Array(w1, w1) -> (w16:dbl[])
  n59 = case shown="False" w19 {
    selector: w19 -> [_ w1116]
    tunnel: [_ w1116] -> _
    tunnel: w34 -> [w215 _]
    tunnel: w33 -> [w222 _]
    tunnel: w6 -> [w221 _]
    tunnel: w32 -> [w216 w1114]
    tunnel: w31 -> [w218 w1113]
    tunnel: w29 -> [w220 _]
    tunnel: [w219 timestamp[] []] -> w25
    tunnel: w20 -> [w217 w1112]
    tunnel: w18 -> [w211 _]
    tunnel: w16 -> [w214 _]
    tunnel: [w213 w1114] -> w15
    tunnel: w14 -> [w212 _]
    tunnel: w12 -> [w210 w1111]
    tunnel: [w209 w1113] -> w11
    tunnel: [w208 w1112] -> w10
    tunnel: [w207 w1111] -> w9
    tunnel: w3 -> [w206 w1110]
    tunnel: [w205 w1110] -> w2
    tunnel: w1 -> [w204 _]
    tunnel: w1 -> [w203 _]
    frame False {
      # "NI 9216"
      # "NI 9207"
      # "CAEN 2"
      # "CAEN 1"
      # "Lakeshore"
      n60 = while {
        shift-right: [w233] -> _
        shift-left: w222 -> [w271]
        shift-right: [w246] -> _
        shift-left: w221 -> [w260]
        shift-right: [w238] -> w219
        shift-left: w220 -> [w268]
        shift-right: [w262] -> w209
        shift-left: w218 -> [w255]
        shift-right: [w264] -> _
        shift-left: w215 -> [w267]
        shift-right: [w261] -> w208
        shift-left: w217 -> [w266]
        shift-right: [w263] -> w213
        shift-left: w216 -> [w265]
        shift-right: [w242] -> _
        shift-left: w211 -> [w257]
        shift-right: [w244] -> _
        shift-left: w211 -> [w258]
        shift-right: [w240] -> _
        shift-left: w214 -> [w256]
        shift-right: [w228] -> _
        shift-left: w212 -> [w254]
        shift-right: [w252] -> w207
        shift-left: w210 -> [w253]
        shift-right: [w250] -> w205
        shift-left: w206 -> [w251]
        shift-right: [w226] -> _
        shift-left: w204 -> [w227]
        shift-right: [w223] -> _
        shift-left: w203 -> [w224]
        stop <- w269 stop-if-true
        # "Email timer"
        # "Alarm timer"
        # "Alarm status"
        # "LakeShore"
        # "9216 x2 (T)"
        # "9207 (V, mA)"
        # "HV supply altered?"
        # "Setpoint"
        # "Anode timing"
        # "Anode timers"
        # "Integrated flow"
        # "Flow"
        # "Flow"
        # "Integrated Flow"
        # "TOBA"
        # "Array of times"
        # "Latest HV read-outs"
        # "Time per cycle (s)"
        # "Cycle number"
        # "HV values: VSet, Vmax, IMax"
        # "HV values"
        # "TOBA"
        n61 = stacked-sequence {
          seq-local: [_ _ w445 _ _ _ _ _ _ _] -> [_ _ _ w615 _ _ _ _ _ _]
          seq-local: ["Time per cycle (s)" _ _ _ _ _ _ _ _ _] -> [_ _ _ _ _ _ w808 _ _ _]
          seq-local: [_ _ w436 _ _ _ _ _ _ _] -> [_ _ _ _ _ _ w810 _ _ _]
          seq-local: [_ w390 _ _ _ _ _ _ _ _] -> [_ _ _ _ w687 w796 _ _ _ _]
          seq-local: [_ _ w439 _ _ _ _ _ _ _] -> [_ _ _ w610 _ _ _ _ _ _]
          seq-local: [_ w383 _ _ _ _ _ _ _ _] -> [_ _ _ _ _ _ w825 _ _ _]
          seq-local: [_ w378 _ _ _ _ _ _ _ _] -> [_ _ _ _ w725 w788 w812 w913 w948 w1035]
          seq-local: [_ w377 _ _ _ _ _ _ _ _] -> [_ _ _ _ w716 w791 w813 w914 w947 w1037]
          seq-local: [_ w365 _ _ _ _ _ _ _ _] -> [_ _ _ _ w723 w790 w811 _ _ _]
          seq-local: [_ _ _ _ _ _ _ w873 _ _] -> [_ _ _ _ _ _ _ _ w950 w1036]
          tunnel: [w297 _ _ _ _ _ _ _ _ _] -> w232
          tunnel: "stop" -> [w296 _ _ _ _ _ _ _ _ _]
          tunnel: w271 -> [w298 w379 w467 _ _ _ _ _ _ _]
          tunnel: w260 -> [_ w380 _ _ w726 _ _ _ _ _]
          tunnel: [_ _ _ _ w703 _ _ _ _ _] -> w247
          tunnel: w268 -> [_ w357 _ _ _ _ _ _ _ _]
          tunnel: w255 -> [_ _ w474 w616 _ _ _ w930 _ _]
          tunnel: w267 -> [_ _ w472 _ _ _ _ _ _ _]
          tunnel: w266 -> [_ _ w471 w611 _ _ _ w929 _ _]
          tunnel: w265 -> [_ w392 _ _ _ _ _ w928 _ _]
          tunnel: [_ w393 _ _ _ _ _ _ _ _] -> w263
          tunnel: [_ _ w436 _ _ _ _ _ _ _] -> w264
          tunnel: [_ _ w453 _ _ _ _ _ _ _] -> w262
          tunnel: [_ _ w450 _ _ _ _ _ _ _] -> w261
          tunnel: [_ _ _ _ w687 _ _ _ _ _] -> w239
          tunnel: w257 -> [_ _ _ _ _ w794 _ _ _ _]
          tunnel: w258 -> [_ _ _ _ _ w795 _ _ _ _]
          tunnel: w256 -> [_ _ _ w617 _ _ _ _ _ _]
          tunnel: [_ _ _ w612 _ _ _ _ _ _] -> w241
          tunnel: w254 -> [_ w386 _ _ _ _ _ _ _ _]
          tunnel: w253 -> [_ w385 _ _ _ _ _ w927 _ _]
          tunnel: [_ w381 _ _ _ _ _ _ _ _] -> w252
          tunnel: [_ _ _ _ _ w793 _ _ _ _] -> w243
          tunnel: [_ _ _ _ _ w792 _ _ _ _] -> w245
          tunnel: w251 -> [_ w364 _ _ _ _ _ w915 _ _]
          tunnel: [_ w359 _ _ _ _ _ _ _ _] -> w250
          tunnel: [_ _ _ _ _ _ _ _ w952 _] -> w228
          tunnel: w227 -> [_ _ _ _ _ _ _ _ w946 _]
          tunnel: [_ _ _ _ _ _ _ _ w944 _] -> w226
          tunnel: w224 -> [_ _ _ _ _ _ _ _ _ w1023]
          tunnel: [_ _ _ _ _ _ _ _ _ w1022] -> w223
          frame #0 {
            # "Temp input channels\ninside detector"
            # "CAEN channel names\nupdater, real-time"
            # "Creates items in the menu rings, for the channel selectors on the phase diagrams;\nAlters the T warning lights."
            # "Also, dumping ground for variables and controls that may be updated during run-time"
            # "CAEN needle gauges\nMin. and Max. ranges"
            # "To view documentation of modules, look for icons that have a \"Descr.\" label near them,\nright-click these and select \"Description and tip\". For example on frame 2, \"High Voltage\",\na \"Quotient and Remainder\" icon on the left-hand side may be checked out, to view the\ndocumentation for the \"Reading Voltages and Currents\" module, which uses that icon."
            # "Time to wait, in between cycles"
            # "If the program is stopped, a final cycle executes without delay."
            # "Waiting for \"interval time\" to have passed, to start new cycle"
            n62 = Increment(x=w298) -> (x+1=w297:i32)
            "Cycle number" <- w297
            n63 = call "Is Value Changed.vim"("value"="Channel Names (CAEN)") -> ("changed or first call?"=w287:bool)
            n64 = call "Is Value Changed.vim"("value"="Specify up to six temperature sensors inside \nthe detector, separated with a comma.\nNumbers only, single commas!") -> ("changed or first call?"=w289:bool)
            n65 = case shown="True" w287 {
              tunnel: "Channel Names (CAEN)" -> [_ w304]
              frame False {
              }
              frame True {
                n66 = Index Array(array=w304) -> (element #1=→"CAEN 1.0":string, element #2=→"CAEN 1.1":string, element #3=→"CAEN 1.2":string, element #4=→"CAEN 1.3":string, element #5=→"CAEN 2.0":string, element #6=→"CAEN 2.1":string, element #7=→"CAEN 2.2 2":string, element #8=→"CAEN 2.3 2":string)  [unwired: 8 in]
                "CAEN Ch. Names" <- w304
                "Channel Names" <- w304
                "Channel Names" <- w304
              }
            }
            n67 = case shown="True" w289 {
              tunnel: "Specify up to six temperature sensors inside \nthe detector, separated with a comma.\nNumbers only, single commas!" -> [_ w314]
              frame False {
              }
              frame True {
                n68 = Bundle("Average", 666) -> (w320:cluster{string, i32})  [unwired: 1 in]
                n69 = Spreadsheet String To Array(delimiter (Tab)=",", format string="%s", spreadsheet string=w314, array type (2D Dbl)=string[] []) -> (array=w323:string[])
                n70 = for {
                  tunnel: w323 -> [w335] mode=indexing
                  tunnel: [w333] -> w322 mode=indexing
                  tunnel: [w332] -> w313 mode=indexing
                  tunnel: [w331] -> w324 mode=indexing
                  n71 = call <vilib>:"Trim Whitespace.vi"("string"=w335) -> ("trimmed string"=w331:string)  [unwired: 1 in]
                  n72 = Scan From String(input string=w331, default 1=0) -> (output 1=w332:i32)  [unwired: 3 in, 3 out]
                  n73 = Bundle("trimmed string"=w331, w332) -> (w333:cluster{"trimmed string":string, i32})  [unwired: 1 in]
                }
                "Det. T." <- w313
                n74 = Build Array (concatenate)(w322, w320) -> (w321:cluster{"trimmed string":string, i32}[])
                n75 = property on="Temperature channel selector" class="Ring (strict)"("StringsAndValues[]"=w321) -> ()  [unwired: 2 in, 2 out]
                n76 = property on="Temperature Channel Selector" class="Ring (strict)"("StringsAndValues[]"=w321) -> ()  [unwired: 2 in, 2 out]
                n77 = Index Array(array=w324) -> (element #1=→"String":string, element #2=→"String 2":string, element #3=→"String 3":string, element #4=→"String 4":string, element #5=→"String 5":string, element #6=→"String 6":string)  [unwired: 6 in]
                n78 = property on="Temperature Channel Selector" class="Ring (strict)"("StringsAndValues[]"=w322) -> ()  [unwired: 2 in, 2 out]
              }
            }
            n79 = local read "Channel Names (9207, ai0:7)"() -> (w285:string[])
            n80 = To Long Integer(number="Detector pressure input:") -> (32bit integer=→"Det.P input #":i32)
            n81 = To Long Integer(number="Flow meter input:") -> (32bit integer=→"Flow input #":i32)
            n82 = call "Is Value Changed.vim"("value"=w285) -> ("changed or first call?"=w286:bool)
            n83 = case shown="True" w286 {
              tunnel: w285 -> [_ w300]
              frame False {
                # ":D"
              }
              frame True {
                n84 = for {
                  tunnel: w300 -> [w303] mode=indexing
                  tunnel: [w301] -> w299 mode=indexing
                  i -> [w302]
                  n85 = Bundle("Or give name if \"Other\""=w303, w302) -> (w301:cluster{"Or give name if \"Other\"":string, i32})  [unwired: 1 in]
                }
                n86 = property on="Detector pressure input:" class="Ring (strict)"("StringsAndValues[]"=w299) -> ()  [unwired: 2 in, 2 out]
                n87 = property on="Flow meter input:" class="Ring (strict)"("StringsAndValues[]"=w299) -> ()  [unwired: 2 in, 2 out]
              }
            }
            n88 = case shown="False" w296 {
              tunnel: "Time per cycle (s)" -> [w352 _]
              frame False {
                n89 = while {
                  tunnel: w352 -> [w354]
                  stop <- w356 stop-if-true
                  n90 = call "Elapsed Time"("Time Target (s)"=w354) -> ("Elapsed Time (s)"=w355:dbl, "Time has Elapsed"=w356:bool)  [unwired: 11 in, 6 out]
                  n91 = Subtract(x=w354, y=w355) -> (x-y=→"Time until next cycle":dbl)
                }
              }
              frame True {
              }
            }
            n92 = stacked-sequence {
              frame #0 {
                n93 = property on="CAEN 1.0" class="Knob (strict)"("Scale.Minimum"="Scale.Range:Minimum", "Scale.Maximum"="Scale.Range:Maximum") -> ()  [unwired: 2 in, 2 out]
                n94 = property on="CAEN 1.1" class="Knob (strict)"("Scale.Minimum"="Scale.Range:Minimum 2", "Scale.Maximum"="Scale.Range:Maximum 2") -> ()  [unwired: 2 in, 2 out]
              }
              frame #1 {
                n95 = property on="CAEN 1.2" class="Knob (strict)"("Scale.Minimum"="Scale.Range:Minimum 3", "Scale.Maximum"="Scale.Range:Maximum 3") -> ()  [unwired: 2 in, 2 out]
                n96 = property on="CAEN 1.3" class="Knob (strict)"("Scale.Maximum"="Scale.Range:Maximum 4", "Scale.Minimum"="Scale.Range:Minimum 4") -> ()  [unwired: 2 in, 2 out]
              }
              frame #2 {
                n97 = property on="CAEN 2.1" class="Knob (strict)"("Scale.Maximum"="Scale.Range:Maximum 6", "Scale.Minimum"="Scale.Range:Minimum 6") -> ()  [unwired: 2 in, 2 out]
                n98 = property on="CAEN 2.0" class="Knob (strict)"("Scale.Maximum"="Scale.Range:Maximum 5", "Scale.Minimum"="Scale.Range:Minimum 5") -> ()  [unwired: 2 in, 2 out]
              }
              frame #3 {
                n99 = property on="CAEN 2.2" class="Knob (strict)"("Scale.Maximum"="Scale.Range:Maximum 7", "Scale.Minimum"="Scale.Range:Minimum 7") -> ()  [unwired: 2 in, 2 out]
                n100 = property on="CAEN 2.3" class="Knob (strict)"("Scale.Maximum"="Scale.Range:Maximum 8", "Scale.Minimum"="Scale.Range:Minimum 8") -> ()  [unwired: 2 in, 2 out]
              }
            }
          }
          frame #1 {
            # "DAQmx Read above will replace dummy data below,\nonce the 9216 modules are functioning"
            # "Descr"
            # "NI 9207 8x V, 8x mA"
            # "Case to ignore runtime errors; unpack later"
            # "Module 1 tasks+status"
            # "Temps (NI)"
            # "9216 T     (NI) x16\n9207 V     (NI)  x8\n9207 mA (NI)  x8\nTemp        (LS)  x2\nHeater %           x1"
            # "Temp A, Temp B, heater power"
            # "Measurements and conversions"
            n101 = case shown="True" "Run lakeshore?" {
              tunnel: [w416 w427] -> w393
              tunnel: w392 -> [w416 w426]
              tunnel: [-273.0 ("Input A") w425] -> w389
              tunnel: [-273.0 ("Input B") w424] -> w388
              tunnel: [73.0 ("Heater 1 (%)") w423] -> w387
              tunnel: w386 -> [_ w421]
              tunnel: [-274.0 "Setpoint (°C)"] -> w383
              frame False {
              }
              frame True {
                # "LS output"
                # "P\nI\nD"
                n102 = Select(t=0, s=w421, f="Heater range") -> (s? t:f=w418:i32)
                n103 = Unbundle("PID settings") -> ("P"=w432:dbl, "I"=w431:dbl, "D"=w430:dbl)
                n104 = Unbundle(w426) -> ("VISA resource name out"=w434:refnum<visa-resource-name>, "error out"=w433:errorcluster)
                n105 = call "Lakeshore subVI.vi"("Setpoint"="Setpoint (°C)", "Rate (D) (X.X %)"=w430, "Range"=w418, "Reset (I) (XX.X)"=w431, "Gain (P) (XX.X)"=w432, "error in (no error)"=w433, "VISA resource name"=w434) -> ("Input B"=w424:dbl, "Input A"=w425:dbl, "error out"=w428:errorcluster, "VISA resource name out"=w429:refnum<visa-resource-name>, "Heater 1 (%)"=w423:dbl)
                n106 = Bundle("VISA resource name out"=w429, "error out"=w428) -> (w427:T3)  [unwired: 1 in]
              }
            }
            n107 = Get Date/Time In Seconds() -> (seconds since 1Jan1904=w391:timestamp)
            n108 = Quotient & Remainder(x=w379, y="Read T every N cycles") -> (x-y*floor(x/y)=w382:i32)  [unwired: 1 out]
            n109 = Unbundle(w364) -> ("task out"=w363:refnum<k21>, "error out"=w362:errorcluster)
            n110 = Build Array (concatenate)(w357, w391) -> (w390:timestamp[])
            n111 = Unbundle(w385) -> ("task out"=w369:refnum<k21>, "error out"=w368:errorcluster)
            n112 = case shown="0" w382 {
              tunnel: w380 -> [_ w409]
              tunnel: [w402 w405] -> w377
              tunnel: w379 -> [w401 _]
              frame 0 {
                # "Dummy data"
                # "New temperatures"
                n113 = Add(x=w401, y=-95.0 ("element")) -> (x+y=w404:dbl)
                n114 = Initialize Array(w404, 16) -> (w402:dbl[])
              }
              frame 1, Default {
                # "Gets 1st 16 Col's\nfrom last row:\nPrevious 16 temps."
                # "Get previous temps"
                n115 = Array Size(array=w409) -> (size(s)=w411:i32[])
                n116 = Index Array(array=w411, index=0) -> (element=w412:i32)
                n117 = Decrement(x=w412) -> (x-1=w408:i32)
                n118 = Index Array(array=w409, index (row)=w408) -> (element=w407:dbl[])  [unwired: 1 in]
                n119 = Array Subset(array=w407, length=16) -> (w405:dbl[])  [unwired: 1 in]
              }
            }
            n120 = call-poly <vilib>:"DAQmx Read.vi"("task/channels in"=w363, "error in"=w362) -> ("task out"=w361:refnum<k21>, "data"=→"Temperatures":dbl[], "error out"=w360:errorcluster)  [unwired: 11 in]
            n121 = call-poly <vilib>:"DAQmx Read.vi"("task/channels in"=w369, "error in"=w368) -> ("task out"=w367:refnum<k21>, "data"=w376:dbl[], "error out"=w366:errorcluster)  [unwired: 11 in]
            "Raw readouts (V, mA)" <- w376
            n122 = Build Array (concatenate)("Offsets\nsubtracted", "Offsets\nsubtracted") -> (w370:dbl[])
            n123 = Build Array (concatenate)("Multipliers", "Multipliers") -> (w373:dbl[])
            n124 = for {
              tunnel: w370 -> [w399] mode=indexing
              tunnel: w376 -> [w398] mode=indexing
              tunnel: w373 -> [w396] mode=indexing
              tunnel: [w395] -> w378 mode=indexing
              n125 = Subtract(x=w398, y=w399) -> (x-y=w397:dbl)
              n126 = Multiply(x=w397, y=w396) -> (x*y=w395:dbl)
            }
            n127 = Bundle("task out"=w361, "error out"=w360) -> (w359:T4)  [unwired: 1 in]
            n128 = Bundle("task out"=w367, "error out"=w366) -> (w381:T4)  [unwired: 1 in]
            n129 = Build Array(w389, w388, w387) -> (w365:dbl[])
            "LakeShore readings" <- w365
            "LakeShore readings 2" <- w365
          }
          frame #2 {
            # "Alter voltages if button clicked"
            # "2"
            # "1"
            # "Descr."
            # "Descr."
            # "VMON1  x4 \nVMON2  x4\nIMON1    x4\nIMON2    x4"
            # "Needle gauge Voltage displays"
            # "1"
            # "2"
            # "1"
            # "2"
            # "Reads new V and A every N cycles,\nor passes previous values"
            # "High Voltage"
            n130 = Unbundle(w474) -> ("VISA resource name out"=w456:refnum<visa-resource-name>, "error out"=w473:errorcluster)
            n131 = Unbundle(w471) -> ("VISA resource name out"=w455:refnum<visa-resource-name>, "error out"=w470:errorcluster)
            n132 = Quotient & Remainder(x=w467, y="Read CAEN units \nevery N cycles") -> (x-y*floor(x/y)=w440:i32)  [unwired: 1 out]
            n133 = Build Array (concatenate)("VSet (V)", "VMax (V)", "IMax (uA)") -> (w445:dbl[])
            n134 = case shown="0" w440 {
              tunnel: w456 -> [w599 _]
              tunnel: w473 -> [w598 w607]
              tunnel: w472 -> [_ w603]
              tunnel: w455 -> [w589 _]
              tunnel: w470 -> [w586 w608]
              tunnel: [w585 w608] -> w457
              tunnel: [w595 w607] -> w458
              tunnel: [w594 w603] -> w436
              tunnel: [w592 w604] -> w469
              tunnel: [w590 w600] -> w468
              frame 0 {
                # "All data x16"
                # "Voltages x8"
                # "Currents x8"
                # "Read"
                n135 = call "READ_SUPPLY.vi"("VISA resource name"=w599, "Board address"=u8 0, "NChannels"=u8 4, "error in (no error)"=w598) -> ("VMon values (V)"=w593:dbl[], "IMon values (uA)"=w591:dbl[], "error out"=w595:errorcluster)  [unwired: 9 in]
                n136 = call "READ_SUPPLY.vi"("VISA resource name"=w589, "Board address"=u8 0, "NChannels"=u8 4, "error in (no error)"=w586) -> ("VMon values (V)"=w584:dbl[], "IMon values (uA)"=w583:dbl[], "error out"=w585:errorcluster)  [unwired: 9 in]
                n137 = Build Array (concatenate)(w591, w583) -> (w590:dbl[])
                n138 = Build Array (concatenate)(w593, w584) -> (w592:dbl[])
                n139 = Build Array (concatenate)(w593, w584, w591, w583) -> (w594:dbl[])
              }
              frame 1, Default {
                # "Don't read: pass previous"
                n140 = Array Subset(array=w603, index=0, length=8) -> (w604:dbl[])
                n141 = Array Subset(array=w603, index=8, length=8) -> (w600:dbl[])
              }
            }
            "Voltages" <- w469
            "Vmon (V)" <- w469
            "IMon (uA)" <- w468
            n142 = Build Array("Apply Voltage", "Set to zero", "Kill voltage") -> (w439:bool[])
            n143 = Search 1D Array(1D array=w439, element=TRUE) -> (index of element=w459:i32)  [unwired: 1 in]
            n144 = case shown="0" w459 {
              tunnel: w458 -> [w491 w525 w558 w579]
              tunnel: w457 -> [w478 w515 w547 w581]
              tunnel: w456 -> [w487 w522 w555 w582]
              tunnel: w455 -> [w476 w513 w545 w580]
              tunnel: [w488 w523 w556 w579] -> w449
              tunnel: [w487 w522 w555 w582] -> w454
              tunnel: [w475 w512 w544 w581] -> w451
              tunnel: [w476 w513 w545 w580] -> w452
              tunnel: "VSet (V)" -> [w485 _ w553 _]
              tunnel: "VMax (V)" -> [w484 w520 _ _]
              tunnel: "IMax (uA)" -> [w483 w519 w552 _]
              frame 0 {
                w477 = 4 ("length")
                w482 = 4 ("length")
                # "Last four"
                # "First four"
                # "Apply voltage"
                n145 = Array Subset(array=w485, length=w482) -> (w490:dbl[])  [unwired: 1 in]
                n146 = Array Subset(array=w484, length=w482) -> (w489:dbl[])  [unwired: 1 in]
                n147 = Array Subset(array=w483, length=w482) -> (w486:dbl[])  [unwired: 1 in]
                n148 = Array Subset(array=w485, index=w477) -> (w481:dbl[])  [unwired: 1 in]
                n149 = Array Subset(array=w484, index=w477) -> (w480:dbl[])  [unwired: 1 in]
                n150 = Array Subset(array=w483, index=w477) -> (w479:dbl[])  [unwired: 1 in]
                n151 = for {
                  tunnel: w487 -> [w510]
                  tunnel: w491 -> [w509]
                  tunnel: w490 -> [w506] mode=indexing
                  tunnel: w489 -> [w504] mode=indexing
                  tunnel: w486 -> [w503] mode=indexing
                  tunnel: [w502] -> w488
                  i -> [w511]
                  n152 = call "SET_SUPPLY_CHANNEL.vi"("VISA resource name"=w510, "Voltage Level (0.0 V)"=w506, "Enable (OFF)"=TRUE, "Board address"=u8 0, "NChannels"=u8 4, "Channel (0)"=w511, "error in (no error)"=w509, "Voltage Max (0.0 V)"=w504, "Current Limit (0.00 uA)"=w503) -> ("error out"=w502:errorcluster)  [unwired: 6 in]
                }
                n153 = for {
                  tunnel: w476 -> [w501]
                  tunnel: w478 -> [w495]
                  tunnel: w481 -> [w500] mode=indexing
                  tunnel: w480 -> [w499] mode=indexing
                  tunnel: w479 -> [w498] mode=indexing
                  tunnel: [w494] -> w475
                  i -> [w497]
                  n154 = call "SET_SUPPLY_CHANNEL.vi"("VISA resource name"=w501, "Voltage Level (0.0 V)"=w500, "Enable (OFF)"=TRUE, "Board address"=u8 0, "NChannels"=u8 4, "Channel (0)"=w497, "error in (no error)"=w495, "Voltage Max (0.0 V)"=w499, "Current Limit (0.00 uA)"=w498) -> ("error out"=w494:errorcluster)  [unwired: 6 in]
                }
              }
              frame 1 {
                w514 = 4 ("length")
                w518 = 4 ("length")
                # "Set V to zero"
                n155 = Array Subset(array=w519, length=w518) -> (w521:dbl[])  [unwired: 1 in]
                n156 = Array Subset(array=w520, length=w518) -> (w524:dbl[])  [unwired: 1 in]
                n157 = Array Subset(array=w520, index=w514) -> (w517:dbl[])  [unwired: 1 in]
                n158 = Array Subset(array=w519, index=w514) -> (w516:dbl[])  [unwired: 1 in]
                n159 = for {
                  tunnel: w522 -> [w542]
                  tunnel: w525 -> [w541]
                  tunnel: w524 -> [w538] mode=indexing
                  tunnel: w521 -> [w537] mode=indexing
                  tunnel: [w536] -> w523
                  i -> [w543]
                  w535 = u8 0 ("Board address")
                  n160 = call "SET_SUPPLY_CHANNEL.vi"("VISA resource name"=w542, "Voltage Level (0.0 V)"=w535, "Enable (OFF)"=TRUE, "Board address"=w535, "NChannels"=u8 4, "Channel (0)"=w543, "error in (no error)"=w541, "Voltage Max (0.0 V)"=w538, "Current Limit (0.00 uA)"=w537) -> ("error out"=w536:errorcluster)  [unwired: 6 in]
                }
                n161 = for {
                  tunnel: w513 -> [w526]
                  tunnel: w515 -> [w531]
                  tunnel: w517 -> [w530] mode=indexing
                  tunnel: w516 -> [w529] mode=indexing
                  tunnel: [w527] -> w512
                  i -> [w532]
                  w534 = 0 ("length")
                  n162 = call "SET_SUPPLY_CHANNEL.vi"("VISA resource name"=w526, "Voltage Level (0.0 V)"=w534, "Enable (OFF)"=TRUE, "Board address"=w534, "NChannels"=u8 4, "Channel (0)"=w532, "error in (no error)"=w531, "Voltage Max (0.0 V)"=w530, "Current Limit (0.00 uA)"=w529) -> ("error out"=w527:errorcluster)  [unwired: 6 in]
                }
              }
              frame 2 {
                w546 = 4 ("length")
                w550 = 2 ("length")
                w551 = 4 ("length")
                # "CAEN 2: Top gate, Bottom gate"
                # "CAEN 1 values:\nPMT1&2, Anode, Cathode"
                # "Set VMax to zero, \"Kill\""
                n163 = Array Subset(array=w552, length=w551) -> (w554:dbl[])  [unwired: 1 in]
                n164 = Array Subset(array=w553, length=w551) -> (w557:dbl[])  [unwired: 1 in]
                n165 = Array Subset(array=w553, index=w546, length=w550) -> (w549:dbl[])
                n166 = Array Subset(array=w552, index=w546, length=w550) -> (w548:dbl[])
                n167 = for {
                  tunnel: w555 -> [w577]
                  tunnel: w558 -> [w576]
                  tunnel: w557 -> [w573] mode=indexing
                  tunnel: w554 -> [w571] mode=indexing
                  tunnel: [w570] -> w556
                  i -> [w578]
                  n168 = call "SET_SUPPLY_CHANNEL.vi"("VISA resource name"=w577, "Voltage Level (0.0 V)"=w573, "Enable (OFF)"=TRUE, "Board address"=u8 0, "NChannels"=u8 4, "Channel (0)"=w578, "error in (no error)"=w576, "Voltage Max (0.0 V)"=u8 0 ("Board address"), "Current Limit (0.00 uA)"=w571) -> ("error out"=w570:errorcluster)  [unwired: 6 in]
                }
                n169 = for {
                  tunnel: w545 -> [w559]
                  tunnel: w547 -> [w562]
                  tunnel: w549 -> [w565] mode=indexing
                  tunnel: w548 -> [w563] mode=indexing
                  tunnel: [w561] -> w544
                  i -> [w568]
                  n170 = call "SET_SUPPLY_CHANNEL.vi"("VISA resource name"=w559, "Voltage Level (0.0 V)"=w565, "Enable (OFF)"=TRUE, "Board address"=u8 0, "NChannels"=u8 4, "Channel (0)"=w568, "error in (no error)"=w562, "Voltage Max (0.0 V)"=0, "Current Limit (0.00 uA)"=w563) -> ("error out"=w561:errorcluster)  [unwired: 6 in]
                }
              }
              frame 3, Default {
                # "\"Executes\" if none of the three buttons have been clicked"
                # "Do nothing"
              }
            }
            n171 = Bundle("VISA resource name out"=w454, "error out"=w449) -> (w453:T3)  [unwired: 1 in]
            n172 = Bundle("VISA resource name out"=w452, "error out"=w451) -> (w450:T3)  [unwired: 1 in]
            n173 = Index Array(array=w436) -> (element #1=→"CAEN 1.0":dbl, element #2=→"CAEN 1.1":dbl, element #3=→"CAEN 1.2":dbl, element #4=→"CAEN 1.3":dbl, element #5=→"CAEN 2.0":dbl, element #6=→"CAEN 2.1":dbl, element #7=→"CAEN 2.2":dbl, element #8=→"CAEN 2.3":dbl)  [unwired: 8 in]
          }
          frame #3 {
            # "Descr."
            # "Reset anode"
            n174 = Or Array Elements(Boolean array=w610) -> (logical OR=w609:bool)
            n175 = case shown="True" "Reset anode\nperiodically?" {
              tunnel: w617 -> [_ w623]
              tunnel: w616 -> [_ w632]
              tunnel: w615 -> [_ w637]
              tunnel: w609 -> [_ w621]
              tunnel: [w618 w622] -> w612
              tunnel: w611 -> [_ w631]
              frame False {
                # "Anode Reset Routine inactive:\nkeep timers up to date so activating\nroutine will correctly initiate the timers."
                n176 = Get Date/Time In Seconds() -> (seconds since 1Jan1904=w620:timestamp)
                n177 = To Double Precision Float(number=w620) -> (double precision float=w619:dbl)
                n178 = Build Array(w619, w619) -> (w618:dbl[])
              }
              frame True {
                # "Descr."
                n179 = case shown="\"CAEN 2\"" "CAEN unit selector" {
                  tunnel: w632 -> [w651 _]
                  tunnel: w631 -> [_ w653]
                  tunnel: [w651 w653] -> w630
                  tunnel: [0 4] -> w628
                  frame "CAEN 1", Default {
                  }
                  frame "CAEN 2" {
                  }
                }
                n180 = call "anode_timing.vi"("Keep off for X seconds"="Keep off for X seconds", "Array of timers"=w623, "Kill every Y minutes"="Kill every Y minutes") -> ("Time to kill"=w639:bool, "Time until reset"=→"Seconds until \nanode reset":dbl, "Time until autokill"=→"Seconds until \nanode autokill":dbl, "Time to reset"=w640:bool)  [unwired: 5 in]
                "Killed" <- w639
                "Restarted" <- w640
                n181 = Add(x=w628, y="Anode ch.") -> (x+y=w626:i32)
                n182 = Build Array(w639, w640, w621) -> (w643:bool[])
                n183 = Add(x=w626, y=8) -> (x+y=w633:i32)
                n184 = Add(x=w626, y=16) -> (x+y=w634:i32)
                n185 = Search 1D Array(1D array=w643, element=TRUE) -> (index of element=w642:i32)  [unwired: 1 in]
                n186 = Unbundle(w630) -> ("VISA resource name out"=w648:refnum<visa-resource-name>, "error out"=w647:errorcluster)
                n187 = Index Array(array=w637, index #1=w626, index #2=w633, index #3=w634) -> (element #1=w646:dbl, element #2=w644:dbl, element #3=w645:dbl)
                n188 = case shown="2" w642 {
                  tunnel: w646 -> [_ w677 _ _]
                  tunnel: w644 -> [w662 w676 _ _]
                  tunnel: w645 -> [w664 w675 _ _]
                  tunnel: w648 -> [w669 w680 _ _]
                  tunnel: w647 -> [w668 w679 _ _]
                  tunnel: "Anode ch." -> [w660 w673 _ _]
                  tunnel: w623 -> [w655 _ _ w686]
                  tunnel: [w654 w670 w683 w686] -> w622
                  frame 0 {
                    # "Set Anode Voltage to zero,\nreset the 1st timer"
                    # "Anode Vset to zero"
                    n189 = Get Date/Time In Seconds() -> (seconds since 1Jan1904=w658:timestamp)
                    n190 = Index Array(array=w655, index=1) -> (element=w656:dbl)
                    n191 = To Double Precision Float(number=w658) -> (double precision float=w657:dbl)
                    n192 = call "SET_SUPPLY_CHANNEL.vi"("VISA resource name"=w669, "Voltage Level (0.0 V)"=0.0, "Enable (OFF)"=TRUE, "Board address"=u8 0, "NChannels"=u8 4, "Channel (0)"=w660, "error in (no error)"=w668, "Voltage Max (0.0 V)"=w662, "Current Limit (0.00 uA)"=w664) -> ("error out"=w663:errorcluster)  [unwired: 6 in]
                    n193 = Build Array(w657, w656) -> (w654:dbl[])
                    n194 = call <vilib>:"Simple Error Handler.vi"("error in (no error)"=w663) -> ()  [unwired: 4 in, 5 out]
                  }
                  frame 1 {
                    # "Set Anode Voltage to defined value,\nreset both timers"
                    # "Anode Vset applied"
                    n195 = Get Date/Time In Seconds() -> (seconds since 1Jan1904=w672:timestamp)
                    n196 = To Double Precision Float(number=w672) -> (double precision float=w671:dbl)
                    n197 = call "SET_SUPPLY_CHANNEL.vi"("VISA resource name"=w680, "Voltage Level (0.0 V)"=w677, "Enable (OFF)"=TRUE, "Board address"=u8 0, "NChannels"=u8 4, "Channel (0)"=w673, "error in (no error)"=w679, "Voltage Max (0.0 V)"=w676, "Current Limit (0.00 uA)"=w675) -> ("error out"=w674:errorcluster)  [unwired: 6 in]
                    n198 = Build Array(w671, w671) -> (w670:dbl[])
                    n199 = call <vilib>:"Simple Error Handler.vi"("error in (no error)"=w674) -> ()  [unwired: 4 in, 5 out]
                  }
                  frame 2 {
                    # "Change Voltage button pressed"
                    # "Reset both timers"
                    n200 = Get Date/Time In Seconds() -> (seconds since 1Jan1904=w685:timestamp)
                    n201 = To Double Precision Float(number=w685) -> (double precision float=w684:dbl)
                    n202 = Build Array(w684, w684) -> (w683:dbl[])
                  }
                  frame 3, Default {
                    # "Timers stay at previous value,\nso difference between those and\ncurrent time keeps incrementing"
                    # "No event"
                  }
                }
              }
            }
            n203 = To Time Stamp(1:w612) -> (0:→"Anode timers":timestamp[])
            "?" <- "Reset anode\nperiodically?"
          }
          frame #4 {
            w705 = 16 ("index")
            # "Plots 9207 output vs time"
            # "Descr."
            # "Moving averages"
            # "Historic graphs: Phase, 9207 ai, Flow, Heater, Temperature"
            # "Non-historic Temperature + Det. Pressure"
            # "Updated TOBA"
            # "Descr."
            # "Latest Detector Pressure"
            # "Plots individual lists of Temp. vs. t"
            # "Plots and moving averages"
            n204 = Build Array (concatenate)(w716, w725, w723) -> (w724:dbl[])
            n205 = Build Array (concatenate)(w726, w724) -> (w703:dbl[][])
            "TOBA appended" <- w703
            n206 = local read "Det. T."() -> (w697:i32[])
            n207 = local read "Flow input #"() -> (w693:i32)
            n208 = local read "Det.P input #"() -> (w694:i32)
            n209 = Equal?(x=666, y="Temperature channel selector") -> (x = y?=w717:bool)
            n210 = case shown="True" w717 {
              tunnel: w716 -> [w759 w765]
              tunnel: w697 -> [_ w764]
              tunnel: [w758 w760] -> w714
              tunnel: "Temperature channel selector" -> [w757 _]
              frame False {
                n211 = Index Array(array=w759, index=w757) -> (element=w758:dbl)
              }
              frame True {
                n212 = for {
                  tunnel: w765 -> [w768]
                  tunnel: w764 -> [w767] mode=indexing
                  tunnel: [w766] -> w761 mode=indexing
                  n213 = Index Array(array=w768, index=w767) -> (element=w766:dbl)
                }
                n214 = Array Size(array=w761) -> (size(s)=w763:i32)
                n215 = Add Array Elements(numeric array=w761) -> (sum=w762:dbl)
                n216 = Divide(x=w762, y=w763) -> (x/y=w760:dbl)
              }
            }
            n217 = Add(x=w694, y=w705) -> (x+y=w707:i32)
            n218 = Add(x=w705, y=w693) -> (x+y=w704:i32)
            n219 = Index Array(array=w703, index (col)=34 ("disabled index (col)")) -> (element=w710:dbl[])  [unwired: 1 in]
            n220 = Index Array(array=w703, index (col) #1=w707, index (col) #2=w704) -> (element #1=w706:dbl[], element #2=w691:dbl[])  [unwired: 2 in]
            n221 = Index Array(array=w703, index (col)="Temperature Channel Selector") -> (element=w712:dbl[])  [unwired: 1 in]
            n222 = local read "Det.P input #"() -> (w695:i32)
            n223 = Bundle(w712, w706) -> (w732:cluster{dbl[], dbl[]})  [unwired: 1 in]
            n224 = for {
              N: 8 -> [_]
              tunnel: w703 -> [w749]
              tunnel: w687 -> [w741]
              tunnel: [w746] -> w701 mode=indexing
              tunnel: [w740] -> w700 mode=indexing
              i -> [w745]
              n225 = Add(x=w745, y=24) -> (x+y=w743:i32)
              n226 = Add(x=16, y=w745) -> (x+y=w748:i32)
              n227 = Index Array(array=w749, index (col) #1=w748, index (col) #2=w743) -> (element #1=w747:dbl[], element #2=w742:dbl[])  [unwired: 2 in]
              n228 = Bundle(w741, w747) -> (w746:cluster{timestamp[], dbl[]})  [unwired: 1 in]
              n229 = Bundle(w741, w742) -> (w740:cluster{timestamp[], dbl[]})  [unwired: 1 in]
            }
            "9207 (ai 0:7, Volts)" <- w701
            "9207 (ai 8:15, Amperes)" <- w700
            n230 = Bundle(w687, w691) -> (w730:cluster{timestamp[], dbl[]})  [unwired: 1 in]
            n231 = Build Array(w730) -> (→"Flow (SLPM)":cluster{timestamp[], dbl[]}[])
            n232 = Index Array(array=w725, index=w695) -> (element=w733:dbl)
            n233 = Build Array(w732) -> (→"Historical Large Phase Diagram":cluster{dbl[], dbl[]}[])
            n234 = Bundle(w714, w733) -> (w737:cluster{dbl, dbl})  [unwired: 1 in]
            n235 = Bundle(w687, w710) -> (w728:cluster{timestamp[], dbl[]})  [unwired: 1 in]
            n236 = Build Array(w737) -> (→"Phase Diagram":cluster{dbl, dbl}[])
            n237 = Build Array(w728) -> (→"Heater power (%)":cluster{timestamp[], dbl[]}[])
            n238 = local read "Det. T."() -> (w696:i32[])
            n239 = Equal?(x=666, y="Temperature Channel Selector") -> (x = y?=w719:bool)
            n240 = call "moving_avg.vi"("N samples"="N samples", "Array"=w706) -> ("Numeric"=→"Detector Pressure":dbl)  [unwired: 9 in]
            n241 = call "moving_avg.vi"("N samples"="N samples", "Array"=w691) -> ("Numeric"=→"Average Flow (SLPM)":dbl)  [unwired: 9 in]
            n242 = for {
              N: 16 -> [_]
              tunnel: w687 -> [w785]
              tunnel: [w784] -> w738 mode=indexing
              tunnel: w703 -> [w783]
              i -> [w782]
              n243 = Index Array(array=w783, index (col)=w782) -> (element=w781:dbl[])  [unwired: 1 in]
              n244 = Bundle(w785, w781) -> (w784:cluster{timestamp[], dbl[]})  [unwired: 1 in]
            }
            "Temperature (ai 0:15, °C)" <- w738
            n245 = case shown="False" w719 {
              tunnel: w716 -> [w771 w777]
              tunnel: w696 -> [_ w776]
              tunnel: [w770 w772] -> w722
              tunnel: "Temperature Channel Selector" -> [w769 _]
              frame False {
                n246 = Index Array(array=w771, index=w769) -> (element=w770:dbl)
              }
              frame True {
                n247 = for {
                  tunnel: w777 -> [w780]
                  tunnel: w776 -> [w779] mode=indexing
                  tunnel: [w778] -> w773 mode=indexing
                  n248 = Index Array(array=w780, index=w779) -> (element=w778:dbl)
                }
                n249 = Array Size(array=w773) -> (size(s)=w775:i32)
                n250 = Add Array Elements(numeric array=w773) -> (sum=w774:dbl)
                n251 = Divide(x=w774, y=w775) -> (x/y=w772:dbl)
              }
            }
            n252 = local read "Channel Names (9207, ai8:15)"() -> (w699:string[])
            n253 = local read "Channel Names (9207, ai0:7)"() -> (w698:string[])
            n254 = call "Is Value Changed.vim"("value"=w699) -> ("changed or first call?"=w708:bool)
            n255 = call "Is Value Changed.vim"("value"=w698) -> ("changed or first call?"=w709:bool)
            n256 = Bundle(w722, w733) -> (w735:cluster{dbl, dbl})  [unwired: 1 in]
            n257 = case shown="True" w708 {
              tunnel: w699 -> [_ w751]
              frame False {
              }
              frame True {
                n258 = for {
                  tunnel: w751 -> [w752] mode=indexing
                  i -> [w753]
                  n259 = property on="9207 (ai 8:15, Amperes)" class="XYGraph (strict)"("Active Plot"=w753, "Plot.Plot Name"=w752) -> ()  [unwired: 2 in, 2 out]
                }
              }
            }
            n260 = case shown="True" w709 {
              tunnel: w698 -> [_ w754]
              frame False {
              }
              frame True {
                n261 = for {
                  tunnel: w754 -> [w755] mode=indexing
                  i -> [w756]
                  n262 = property on="9207 (ai 0:7, Volts)" class="XYGraph (strict)"("Active Plot"=w756, "Plot.Plot Name"=w755) -> ()  [unwired: 2 in, 2 out]
                }
              }
            }
            n263 = Build Array(w735) -> (→"Large Phase Diagram":cluster{dbl, dbl}[])
          }
          frame #5 {
            # "Temp A, Temp B, Heater%"
            # "Temperatures x16\nTo indicators on the physical schematic"
            # "Individual latest 9207 readings.\nIndicators go here. Array is 1x16,\nitems have been converted using\nthe offsets and multipliers"
            # "Displays"
            n264 = local read "Flow input #"() -> (w789:i32)
            n265 = case shown="False" "Reset?" {
              tunnel: [w801 0.0] -> w797
              tunnel: w794 -> [w801 _]
              frame False {
              }
              frame True {
              }
            }
            n266 = Index Array(array=w788) -> ()  [unwired: 16 in, 16 out]
            n267 = Index Array(array=w788, index=w789) -> (element=w792:dbl)
            n268 = call "Average_flow_x_time.vi"("Array of timestamps"=w796, "Previous Flow"=w795, "Latest Flow"=w792) -> ("Volume (SL)"=w798:dbl)  [unwired: 8 in]
            n269 = case shown="False" "Pause?" {
              tunnel: w797 -> [w805 w806]
              tunnel: w798 -> [w804 _]
              tunnel: [w803 w806] -> w793
              frame False {
                n270 = Add(x=w804, y=w805) -> (x+y=w803:dbl)
              }
              frame True {
              }
            }
            "Integrated Flow (SL)" <- w793
            n271 = Index Array(array=w790) -> (element #1=→"Coldhead" →"Temp A":dbl, element #2=→"Heater" →"Temp B":dbl)  [unwired: 3 in, 1 out]
            n272 = Index Array(array=w791) -> ()  [unwired: 16 in, 16 out]
            "9207 (V; A) Converted" <- w788
            "9216 #1 (°C)" <- w791
            "9216 #2 (°C)" <- w791
          }
          frame #6 {
            # "The same order applies to the headers re-saved,\nbut with an additional line, stating the date/time"
            # "-----------DATA SAVED----------\nHuman-readable timestamp  ;\nTemperatures (16),  2xNI 9216;\nVolts, Amps  (8 x2),     NI 9207;\nTemperature (2),    Lakeshore;\nHeater power (1),  Lakeshore;\nSetpoint (1),           Lakeshore;\nHV readouts (16)          CAEN ;\nCurrent time (s)                ---   ;\nCycle time (s)                    ---   ;"
            # "Saving data"
            n273 = Get Date/Time In Seconds() -> (seconds since 1Jan1904=w824:timestamp)
            n274 = To Double Precision Float(number=w824) -> (double precision float=w809:dbl)
            n275 = Build Array (concatenate)(w813, w812, w811, w825, w810, w809, w808) -> (w823:dbl[])
            n276 = Get Date/Time String() -> (date string=w817:string)  [unwired: 3 in, 1 out]
            n277 = case shown="True" "Re-save headers" {
              frame False {
                # "Just sit around and feel pretty"
              }
              frame True {
                w833 = ""
                # "Append line of most recent channel names to header file"
                n278 = local read "Channel Names (CAEN)"() -> (w832:string[])
                n279 = local read "Channel Names (9207, ai0:7)"() -> (w840:string[])
                n280 = for {
                  N: 16 -> [_]
                  shift-right: [w865] -> w836
                  shift-left: "" -> [w866]
                  i -> [w870]
                  n281 = Format Into String(initial string="t", w870) -> (resulting string=w868:string)  [unwired: 2 in, 1 out]
                  n282 = Concatenate Strings(w866, w868, "\t") -> (w865:string)
                }
                n283 = for {
                  shift-right: [w863] -> w838
                  shift-left: w833 -> [w864]
                  tunnel: w840 -> [w861] mode=indexing
                  n284 = Concatenate Strings(w864, w861, "\t") -> (w863:string)
                }
                n285 = local read "Channel Names (9207, ai8:15)"() -> (w839:string[])
                n286 = for {
                  tunnel: w832 -> [w855] mode=indexing
                  shift-right: [w853] -> w827
                  shift-left: w833 -> [w852]
                  n287 = Concatenate Strings(w852, w855, " (V)", "\t") -> (w853:string)
                }
                n288 = for {
                  shift-right: [w859] -> w835
                  shift-left: w838 -> [w860]
                  tunnel: w839 -> [w857] mode=indexing
                  n289 = Concatenate Strings(w860, w857, "\t") -> (w859:string)
                }
                n290 = for {
                  tunnel: w832 -> [w850] mode=indexing
                  shift-right: [w848] -> w831
                  shift-left: w827 -> [w847]
                  n291 = Concatenate Strings(w847, w850, " (I)", "\t") -> (w848:string)
                }
                n292 = Get Date/Time String() -> (date string=w845:string)  [unwired: 3 in, 1 out]
                n293 = Format Date/Time String() -> (date/time string=w826:string)  [unwired: 3 in]
                n294 = Build Path(base path=path "D:/Log_data/SC_LOG_HEADERS", name or relative path=w845) -> (appended path=w844:path)
                n295 = Concatenate Strings("Time\t", w836, w835, "Temp A\tTemp B\tHeater Power\tSetpoint\t", w831, "Time in seconds\tTime per cycle\t", w826, "\r\n") -> (w828:string)
                n296 = call <vilib>:"Write Spreadsheet String.vi"("append to file? (new file:F)"=TRUE, "spreadsheet string"=w828, "file path (dialog if empty)"=w844) -> ()  [unwired: 7 in, 2 out]
              }
            }
            n297 = Build Path(base path=path "D:/Log_data/SC_LOG", name or relative path=w817) -> (appended path=w816:path)
            n298 = Format Date/Time String() -> (date/time string=w821:string)  [unwired: 3 in]
            n299 = Array To Spreadsheet String(array=w823, 3:"%.3f" ("format string")) -> (spreadsheet string=w819:string)  [unwired: 1 in]
            n300 = Concatenate Strings(w821, "\t", w819) -> (w815:string)
            n301 = call <vilib>:"Write Spreadsheet String.vi"("append to file? (new file:F)"=TRUE, "spreadsheet string"=w815, "file path (dialog if empty)"=w816) -> ()  [unwired: 7 in, 2 out]
          }
          frame #7 {
            # "Status is True if ANY (armed)\ncondition is met"
            # "Detector P. Alert"
            # "Uninteruptable\n Power Supply Alert"
            # "Temp. Warning"
            # "Arms"
            # "Comm. Alert"
            # "Temperature Alert"
            # "Alarm conditions (Temp)"
            # "Check Alarms and Warnings"
            n302 = Unbundle By Name(w915) -> ("error out.status"=w896:bool)
            "NI mod 2&3 status" <- w896
            n303 = Unbundle By Name(w928) -> ("error out.status"=w926:bool)
            "LakeShore status" <- w926
            n304 = Unbundle By Name(w930) -> ("error out.status"=w925:bool)
            "CAEN 1 status" <- w925
            n305 = Unbundle By Name(w929) -> ("error out.status"=w924:bool)
            "CAEN 2 status" <- w924
            n306 = Unbundle By Name(w927) -> ("error out.status"=w923:bool)
            "NI mod1 (P) status" <- w923
            n307 = Build Array(w926, w925, w924, w923, w896) -> (w897:bool[])
            n308 = Build Array("LakeShore", "CAEN 1", "CAEN 2", "NI mod 2&3", "NI mod 1") -> (w892:bool[])
            n309 = call "check_ups.vi"() -> ("Error: no voltages read"=w876:bool, "Timestamp last measured"=→"Timestamp last \nmeasured (UPS)":timestamp, "Minimum input voltage measured"=w886:dbl)  [unwired: 8 in, 1 out]
            "Minimum input voltage measured" <- w886
            n310 = property on="Det.P input #" class="DigNum (strict)"() -> ("Value"=w912:i32)  [unwired: 2 in, 2 out]
            n311 = Or Array Elements(Boolean array=w897) -> (logical OR=→"Comm. status":bool)
            n312 = for {
              tunnel: w897 -> [w933] mode=indexing
              tunnel: w892 -> [w932] mode=indexing
              tunnel: [w931] -> w891 mode=indexing
              n313 = And(x=w933, y=w932) -> (x .and. y?=w931:bool)
            }
            n314 = Index Array(array=w913, index=w912) -> (element=w909:dbl)
            n315 = Less?(x=w886, y="UPS Voltage \nLower Threshold") -> (x < y?=w878:bool)
            n316 = Equal?(x=w886, y=-1.0) -> (x = y?=w877:bool)
            n317 = Less?(x=w909, y="Underpressure threshold") -> (x < y?=w907:bool)
            n318 = Build Array(w878, w877, w876) -> (w875:bool[])
            n319 = Or Array Elements(Boolean array=w891) -> (logical OR=w881:bool)
            n320 = Greater?(x=w909, y="Overpressure threshold") -> (0:w908:bool)
            n321 = Or(x=w908, y=w907) -> (x .or. y?=w906:bool)
            "Det. P. warning" <- w906
            n322 = Or Array Elements(Boolean array=w875) -> (logical OR=w874:bool)
            "Warning" <- w874
            n323 = And(x="UPS", y=w874) -> (x .and. y?=w880:bool)
            n324 = And(x=w906, y="Detector Pressure") -> (x .and. y?=w882:bool)
            n325 = local read "Det. T."() -> (w872:i32[])
            n326 = Build Array("T 1", "T 2", "T 3", "T 4", "T 5", "T 6") -> (w871:bool[])
            n327 = for {
              tunnel: w914 -> [w943]
              tunnel: w872 -> [w942] mode=indexing
              tunnel: w871 -> [w936] mode=indexing
              tunnel: [w935] -> w883 mode=indexing
              tunnel: [w934] -> w898 mode=indexing
              n328 = Index Array(array=w943, index=w942) -> (element=w939:dbl)
              n329 = Less?(x=w939, y="Low Temp threshold") -> (x < y?=w938:bool)
              n330 = Greater?(x=w939, y="High Temp threshold") -> (0:w937:bool)
              n331 = Or(x=w938, y=w937) -> (x .or. y?=w934:bool)
              n332 = And(x=w936, y=w934) -> (x .and. y?=w935:bool)
            }
            n333 = Index Array(array=w898) -> (element #1=→"Boolean":bool, element #2=→"Boolean 2":bool, element #3=→"Boolean 3":bool, element #4=→"Boolean 4":bool, element #5=→"Boolean 5":bool, element #6=→"Boolean 6":bool)  [unwired: 6 in]
            n334 = Build Array (concatenate)(w883, w882, w881, w880) -> (w879:bool[])
            n335 = Or Array Elements(Boolean array=w879) -> (logical OR=w873:bool)
            "Alarm state" <- w873
          }
          frame #8 {
            # "Testing alarm will not interfere"
            # "Act on alarm"
            n336 = Or(x="Test alarm", y=w950) -> (x .or. y?=w951:bool)
            n337 = case shown="True" w951 {
              tunnel: "Test alarm" -> [_ w958]
              tunnel: w948 -> [_ w966]
              tunnel: w947 -> [_ w965]
              tunnel: w946 -> [w954 w956]
              tunnel: "Alarm\nMaster switch" -> [_ w963]
              tunnel: [w954 w957] -> w944
              frame False {
                # "Timer stays at previous value"
              }
              frame True {
                n338 = Get Date/Time In Seconds() -> (seconds since 1Jan1904=w970:timestamp)
                n339 = case shown="True" "\"Sound\" alarm" {
                  frame False {
                  }
                  frame True {
                    n340 = call <vilib>:"Beep.vi"("duration (msec)"=u32 1000, "frequency (Hz)"="Sound alarm\nFrequency (Hz)") -> ()  [unwired: 10 in]
                  }
                }
                n341 = To Double Precision Float(number=w970) -> (double precision float=w967:dbl)
                n342 = Multiply(x="Repeat Alarm SMS\nevery N minutes", y=60.0) -> (x*y=w959:dbl)
                n343 = Subtract(x=w967, y=w956) -> (x-y=w962:dbl)
                n344 = Greater?(x=w962, y=w959) -> (0:w964:bool)
                n345 = And(x=w963, y=w964) -> (x .and. y?=w961:bool)
                n346 = Or(x=w958, y=w961) -> (x .or. y?=w960:bool)
                n347 = case shown="True" w960 {
                  tunnel: w958 -> [_ w985]
                  tunnel: w966 -> [_ w993]
                  tunnel: w965 -> [_ w981]
                  tunnel: [w973 w983] -> w957
                  tunnel: w956 -> [w973 w982]
                  frame False {
                    # "Alarm not armed, or defined time has not yet passed"
                  }
                  frame True {
                    # "Average T in Det."
                    n348 = local read "Det. T."() -> (w999:i32[])
                    n349 = local read "Det.P input #"() -> (w1000:i32)
                    n350 = case shown="True" w985 {
                      tunnel: ["Error encountered inXAMS! Status:" "TESTING the XAMS alarm. Status:"] -> w992
                      tunnel: [w1004 w1007] -> w983
                      tunnel: w982 -> [_ w1007]
                      frame False {
                        n351 = Get Date/Time In Seconds() -> (seconds since 1Jan1904=w1005:timestamp)
                        n352 = To Double Precision Float(number=w1005) -> (double precision float=w1004:dbl)
                      }
                      frame True {
                      }
                    }
                    n353 = for {
                      tunnel: w981 -> [w1018]
                      tunnel: w999 -> [w1014] mode=indexing
                      tunnel: [w1017] -> w998 mode=indexing
                      tunnel: [w1015] -> w976 mode=indexing
                      n354 = Index Array(array=w1018, index=w1014) -> (element=w1017:dbl)
                      n355 = Format Into String(format string="%.0f", w1014) -> (resulting string=w1012:string)  [unwired: 2 in, 1 out]
                      n356 = Format Into String(format string="%.1f", w1017) -> (resulting string=w1010:string)  [unwired: 2 in, 1 out]
                      n357 = Concatenate Strings("\n" ("format string"), w1012, "     " ("format string"), w1010) -> (w1015:string)
                    }
                    n358 = Index Array(array=w993, index=w1000) -> (element=w994:dbl)
                    n359 = Array Size(array=w998) -> (size(s)=w996:i32)
                    n360 = Add Array Elements(numeric array=w998) -> (sum=w997:dbl)
                    n361 = Format Into String(format string="%.3f", w994) -> (resulting string=w988:string)  [unwired: 2 in, 1 out]
                    n362 = Divide(x=w997, y=w996) -> (x/y=w986:dbl)
                    n363 = Format Date/Time String() -> (date/time string=w990:string)  [unwired: 3 in]
                    n364 = Format Into String(format string="%.2f", w986) -> (resulting string=w974:string)  [unwired: 2 in, 1 out]
                    n365 = Concatenate Strings(w992, "\nDate/time: ", w990, "\nDetector Pressure: ", w988, " bar", "\nDetector Temperatures (°C):", "\nCh:   Temp:" ("format string"), w976, "\nAverage detector temperature: ", w974) -> (w980:string)
                    "Alarm (or test) message" <- w980
                    n366 = for {
                      tunnel: w980 -> [w1003]
                      tunnel: "Phone numbers" -> [w1002] mode=indexing
                      n367 = call "send_sms.vi"("Message content"=w1003, "Phone number"=w1002) -> ("standard error"=→"SMS error":string)  [unwired: 8 in, 1 out]
                    }
                  }
                }
              }
            }
            n368 = And(x="Shut off heater \nif Alarm is active", y=w950) -> (x .and. y?=w952:bool)
            "Alarm active 2" <- "Alarm\nMaster switch"
          }
          frame #9 {
            # "Daily e-mail"
            n369 = Get Date/Time In Seconds() -> (seconds since 1Jan1904=w1031:timestamp)
            n370 = To Double Precision Float(number=w1031) -> (double precision float=w1030:dbl)
            n371 = Get Date/Time String(want seconds? (F)=FALSE) -> (time string=w1033:string)  [unwired: 2 in, 1 out]
            n372 = Subtract(x=w1030, y=w1023) -> (x-y=w1029:dbl)
            n373 = Equal?(x=w1033, y="Send status email at time:") -> (x = y?=w1026:bool)
            n374 = Greater?(x=w1029, y=62) -> (0:w1025:bool)
            n375 = Build Array("Send daily email?", w1026, w1025) -> (w1024:bool[])
            n376 = And Array Elements(Boolean array=w1024) -> (logical AND=w1020:bool)
            n377 = Or(x="Send status email now", y=w1020) -> (x .or. y?=w1021:bool)
            n378 = case shown="True" w1021 {
              tunnel: w1037 -> [_ w1072]
              tunnel: w1036 -> [_ w1055]
              tunnel: w1035 -> [_ w1064]
              tunnel: w1023 -> [w1038 _]
              tunnel: [w1038 w1050] -> w1022
              frame False {
              }
              frame True {
                # "Average T in Det."
                n379 = local read "Det. T."() -> (w1073:i32[])
                n380 = Not Equal To 0?(x="Number of Bonus lines") -> (x != 0?=w1043:bool)
                n381 = case shown="False" w1043 {
                  tunnel: [w1078 w1081] -> w1044
                  tunnel: "Number of Bonus lines" -> [_ w1084]
                  frame False {
                    n382 = Build Array("\n[Flavor text module inactive]") -> (w1078:string[])
                  }
                  frame True {
                    n383 = Build Path(base path=path "C:/Users/xams/Desktop/New XAMS Slow Control", name or relative path="cool_beans.txt") -> (appended path=w1085:path)
                    n384 = call-poly <vilib>:"Read Delimited Spreadsheet.vi"("file path (dialog if empty)"=w1085) -> ("all rows"=w1088:string[][])  [unwired: 9 in, 5 out]
                    n385 = Array Size(array=w1088) -> (size(s)=w1090:i32[])
                    n386 = Index Array(array=w1090) -> (element=w1089:i32)  [unwired: 1 in]
                    n387 = for {
                      N: w1084 -> [_]
                      tunnel: w1089 -> [w1095]
                      tunnel: w1088 -> [w1094]
                      tunnel: [w1091] -> w1082 mode=indexing
                      n388 = Random Number (0-1)() -> (number: 0 to 1=w1098:dbl)
                      n389 = Multiply(x=w1095, y=w1098) -> (x*y=w1097:dbl)
                      n390 = Round To Nearest(number=w1097) -> (nearest integer value=w1096:dbl)
                      n391 = Index Array(array=w1094, index (row)=w1096) -> (element=w1092:string[])  [unwired: 1 in]
                      n392 = Concatenate Strings("\n", w1092) -> (w1091:string)
                    }
                    n393 = Concatenate Strings("\n\nBy the way, did you know?", w1082) -> (w1080:string)
                    n394 = Build Array(w1080) -> (w1081:string[])
                  }
                }
                n395 = local read "Det.P input #"() -> (w1065:i32)
                n396 = for {
                  tunnel: w1073 -> [w1107] mode=indexing
                  tunnel: [w1108] -> w1057 mode=indexing
                  tunnel: w1072 -> [w1101]
                  tunnel: [w1100] -> w1071 mode=indexing
                  n397 = Index Array(array=w1101, index=w1107) -> (element=w1100:dbl)
                  n398 = Format Into String(format string="%.0f", w1107) -> (resulting string=w1104:string)  [unwired: 2 in, 1 out]
                  n399 = Format Into String(format string="%.2f", w1100) -> (resulting string=w1102:string)  [unwired: 2 in, 1 out]
                  n400 = Concatenate Strings("\nCh: " ("format string"), w1104, ", Temp: " ("format string"), w1102, "°C." ("format string")) -> (w1108:string)
                }
                n401 = Array Size(array=w1071) -> (size(s)=w1076:i32)
                n402 = Add Array Elements(numeric array=w1071) -> (sum=w1077:dbl)
                n403 = Index Array(array=w1064, index=w1065) -> (element=w1062:dbl)
                n404 = Divide(x=w1077, y=w1076) -> (x/y=w1074:dbl)
                n405 = Format Into String(format string="%.3f", w1062) -> (resulting string=w1060:string)  [unwired: 2 in, 1 out]
                n406 = Format Into String(format string="%.2f", w1074) -> (resulting string=w1054:string)  [unwired: 2 in, 1 out]
                n407 = Select(t="ACTIVE!!!!!", s=w1055, f="inactive.") -> (s? t:f=w1067:string)
                n408 = Concatenate Strings("Hello, XAMS teammembers.", "\n\nThe alarm is currently ", w1067, "\n\nThe latest detector pressure is: ", w1060, " bar." ("format string"), "\nTemperatures inside the detector are:", w1057, "\nThe average detector temperature is ", w1054, "°C." ("format string"), "\n\nThank you for doing your best today, once again!\nRegards, SC.", w1044) -> (w1049:string)
                "Status email preview" <- w1049
                n409 = call "custom_email_program.vi"("mail server"="smtp.nikhef.nl", "return address"="return address", "message"=w1049, "subject ([No Subject])"="XAMS daily status email.", "Email Adresses"="Email Addresses") -> ("error out"=w1041:errorcluster)  [unwired: 6 in]
                n410 = Unbundle By Name(w1041) -> ("code"=→"Email error":i32, "source"=→"source":string)
                n411 = Get Date/Time In Seconds() -> (seconds since 1Jan1904=w1051:timestamp)
                n412 = To Double Precision Float(number=w1051) -> (double precision float=w1050:dbl)
              }
            }
          }
        }
        n413 = Decrement(x="Cycles to execute") -> (x-1=w249:dbl)
        n414 = Decrement(x=w249) -> (x-1=w248:dbl)
        n415 = Greater?(x=w232, y=w248) -> ()  [unwired: 1 out]
        n416 = Decrement(x="Clear data every N cycles") -> (x-1=w229:dbl)
        n417 = Greater?(x=w232, y=w229) -> (0:w231:bool)
        n418 = And(x="Auto-clear data?", y=w231) -> (x .and. y?=w234:bool)
        n419 = Or(x=w234, y="Clear data") -> (x .or. y?=w236:bool)
        n420 = case shown="False" w236 {
          tunnel: w247 -> [w277 _]
          tunnel: [w277 dbl[][] []] -> w246
          tunnel: w245 -> [w276 _]
          tunnel: [w276 w283] -> w244
          tunnel: w243 -> [w275 _]
          tunnel: [w275 w283] -> w242
          tunnel: w241 -> [w274 _]
          tunnel: [w274 w281] -> w240
          tunnel: w239 -> [w273 _]
          tunnel: [w273 w279] -> w238
          tunnel: w232 -> [w272 _]
          tunnel: [w272 0] -> w233
          frame False {
          }
          frame True {
            w283 = 0.0
            n421 = Get Date/Time In Seconds() -> (seconds since 1Jan1904=w280:timestamp)
            n422 = To Double Precision Float(number=w280) -> (double precision float=w282:dbl)
            n423 = Build Array(w280) -> (w279:timestamp[])
            n424 = Build Array(w282, w282) -> (w281:dbl[])
          }
        }
        n425 = Or(x=FALSE, y="stop") -> (x .or. y?=w269:bool)
        "Auto-clear" <- "Auto-clear data?"
      }
    }
    frame True {
    }
  }
  n426 = flat-sequence {
    tunnel: w15 -> [w1145]
    tunnel: w11 -> [w1136]
    tunnel: w10 -> [w1133]
    tunnel: w9 -> [w1128]
    tunnel: w2 -> [w1117]
    frame #0 {
      w1141 = u16 2 items=["1"=1, "2"=2] ("Heater Output (1:1)")
      w1142 = u16 0 items=["Off", "Low (On)", "Medium", "High"] ("Range (0:Off)")
      # "Important icons! Always press STOP button when done, \notherwise these don't get executed"
      # "Turn off heater, shutdown COM"
      # "Error Handling and Post-Processing (EHaPP)"
      n427 = Unbundle(w1145) -> ("VISA resource name out"=w1144:refnum<visa-resource-name>, "error out"=w1143:errorcluster)
      n428 = Unbundle(w1136) -> ("VISA resource name out"=w1135:refnum<visa-resource-name>, "error out"=w1134:errorcluster)
      n429 = Unbundle(w1133) -> ("VISA resource name out"=w1132:refnum<visa-resource-name>, "error out"=w1131:errorcluster)
      n430 = Unbundle(w1128) -> ("task out"=w1126:refnum<k21>, "error out"=w1124:errorcluster)
      n431 = Unbundle(w1117) -> ("task out"=w1121:refnum<k21>, "error out"=w1119:errorcluster)
      n432 = call <vilib>:"DAQmx Stop Task.vi"("task/channels in"=w1126, "error in"=w1124) -> ("task out"=w1125:refnum<k21>, "error out"=w1123:errorcluster)  [unwired: 12 in]
      n433 = call <vilib>:"DAQmx Stop Task.vi"("task/channels in"=w1121, "error in"=w1119) -> ("task out"=w1120:refnum<k21>, "error out"=w1118:errorcluster)  [unwired: 12 in]
      n434 = call <instrlib>:"Configure Output Range and Manual Value.vi"("VISA resource name"=w1144, "Heater Output (1:1)"=w1141, "Range (0:Off)"=w1142, "Manual Output (0.00 %)"=0.0, "error in (no error)"=w1143) -> ("VISA resource name out"=w1139:refnum<visa-resource-name>, "error out"=w1138:errorcluster)  [unwired: 9 in]
      n435 = call <instrlib>:"Close.vi"("error in (no error)"=w1134, "VISA resource name"=w1135) -> ("error out"=w1130:errorcluster)  [unwired: 9 in]
      n436 = call <instrlib>:"Close.vi"("error in (no error)"=w1131, "VISA resource name"=w1132) -> ("error out"=w1129:errorcluster)  [unwired: 9 in]
      n437 = call <instrlib>:"Close.vi"("error in (no error)"=w1138, "VISA resource name"=w1139) -> ("error out"=w1137:errorcluster)  [unwired: 9 in]
      n438 = call <vilib>:"DAQmx Clear Task.vi"("task in"=w1125, "error in"=w1123) -> ("error out"=w1127:errorcluster)  [unwired: 13 in]
      n439 = call <vilib>:"DAQmx Clear Task.vi"("task in"=w1120, "error in"=w1118) -> ("error out"=w1122:errorcluster)  [unwired: 13 in]
      n440 = call <vilib>:"Simple Error Handler.vi"("error in (no error)"=w1137) -> ()  [unwired: 4 in, 5 out]
      n441 = call <vilib>:"Simple Error Handler.vi"("error in (no error)"=w1130) -> ()  [unwired: 4 in, 5 out]
      n442 = call <vilib>:"Simple Error Handler.vi"("error in (no error)"=w1129) -> ()  [unwired: 4 in, 5 out]
      n443 = call <vilib>:"Simple Error Handler.vi"("error in (no error)"=w1127) -> ()  [unwired: 4 in, 5 out]
      n444 = call <vilib>:"Simple Error Handler.vi"("error in (no error)"=w1122) -> ()  [unwired: 4 in, 5 out]
    }
  }
  n445 = Array Size(array=w25) -> (size(s)=w28:i32)
  n446 = Decrement(x=w28) -> (x-1=w27:i32)
  n447 = Index Array(array=w25, index #1=w27, index #2=1 ("index")) -> (element #1=w26:timestamp, element #2=w7:timestamp)
  n448 = To Double Precision Float(number=w26) -> (double precision float=w24:dbl)
  n449 = To Double Precision Float(number=w7) -> (double precision float=w23:dbl)
  n450 = Subtract(x=w24, y=w23) -> ()  [unwired: 1 out]
  "Started up?" <- w19
